vi "cm2nm_sample_organizer.vi"() -> ()   [LabVIEW 2011]
doc: "Program Purpose:\nThis program has been designed to assist with the tracking of a sample from one analytical instrument to another such as SEM, microscopes, micro x-ray diffraction and other instruments where particular positions/locations on the sample are examined, photographed, etc. The software is designed to easily enter the position of fiducials and locations of interest such that in a future session in the same of different instrument the positions of interest can be re-found through using the known location fiducials in the current and reference session to transform the point into the current sessions coordinate system. The software is dialog box driven guiding the user through the necessary data entry and program choices. Information is stored in a series of text based extensible markup language (XML) files.\n\nSome terminology used for the software:\nSample -- The item itself usually a new standard sample holder designed to have built in fiducials. \nSession -- a particular use the sample in an instrument where the sample is stationary in the instrument so the fiducials only need to be found once to associate it with reference a session. A reference session is a previous session where the fiducials and other spots of interest.\nSpots -- a location or position on the sample where data is taken as an image, spectra or other data forms applicable to analytical instruments. Note fiducials are special spots that are used as references for registering the locations from one session to another.\n\nProgram Startup:\nThe software is designed to be built into a standard windows or OS-X installer by the development platform. Once installed the program will be found under Start->Programs->cm2nm->Sample Organizer or in the OS-x Applications folder. The program will launch and show a graphical uses interface with organized into several selectable tabs. In addition there are developer information tab that will generally hidden from the users:\n• Sample Information\n• LocationDataBase\n• Current Session\n• Plots\n• Current Session Spot Text \n• Transformation Matrix [hidden from users]\nThe software is event driven and will initialize with no session loaded and the buttons to load. There are several buttons available outside the tabs that are of global use:\n• New Sample – press to start with a blank sample. Warnings should are issued about opening a new sample when an old sample may be open, giving operator an opportunity to stop and save. A dialog for entering basic sample information opens when this button is pressed.\n• Load Existing Sample – press to select an exiting sample file. A standard file system dialog box is started allowing user to select a sample file.\n• Save – ensures the current sample data base has been written to the sample file.\n• New Session with this Sample – initiates a new blank session with no spots for the current sample. The new session becomes the current session. A dialog box is started to prompt user for session information. Software will provide ample locations for user to enter notes about the session.\n• Build Date – this is a read only field to allow user to know the version of the software by build date. \n\nBasic File Structure:\n <sample>.xml [top level file that contains an array of pointers to the session data files]\n <session_n>.xml [session information with an array of spots]\n Array of spots has fields that point to files that are generated out side this program either instrument or user generated files associated with spots.\nTabs\nSample Information Tab\nThe sample information tab provides the user with an interface to get an overview of the sample including the sample name or ID and general notes on the sample. This tab has a read only field to provide the file name and path for the sample main database (XML) file. This tab also provides the ability to select a session and spot location for editing or viewing of the information about the sample. The user will use a drop down box containing the session names for the sample. When the users changes the selection on this drop down box the information displayed in the Session Information View field. Another drop down will contain the names of the spots in the selected session. When the user selects the spot the details of that spot will allows be displayed in the Information View window.\n\nLocation Data Base Tab\nThe location data base tab provides a read only overview of the session and spots associated with this sample. Session names are listed on the top row. Spot names are listed in the first column. The table shows X in the boxes at the intersection of a session and spot when a spot was recorded for that session. A C indicates that the position for that spot. The intent is an overview of the data available for the sample.\n\nCurrent Session Tab\nThe current session tab is the primary interface while a sample is in an instrument. The current session tab provides the interface to give status of the session with regards to the number of fiducials found and the current list of spots in the session. A similar view to that in the Sample Information Tab shows the general session information for the current session and the details of a spot selected with a drop down selector. A Modify button allows a user to alter the information about a selected spot through a dialog box driven process. The user is allowed to add new spots and fiducial spots at any time during the session. Another button for Find a Spot From a Previous Session becomes available only after a minimum number of three matching fiducials are first added. A Fiducial Count indicator gives feedback to the user of the number of fiducials located with the number of squares. The color of the squares indicates with yellow that not enough fiducials are been found, blue that a minimum number of fiducials have been found and green when the more than enough have been added. Each of the add spot buttons will open a dialog box to guide the user through the process of the particular type of add.\n\nPlots Tab\nThe Plots Tab will display a graphically X-Y plot of the current constellation of the spots in the current session. Only preliminary development has occurred on this user information screen to date.\n\nCurrent Session Spot Text Tab\nThe Current Session Spot Text provides a text field with a comma delimited output of the spots in the current session with the locations and names of the spots. It is intended for easy pasting into a spreadsheet.\n\nTransfomration Matrix Tab\nThe Transformation Matrix Tab is not intended for general use. It is available in the developers interface for inspection of the coordinate transformation information and a platform to generate some testing information for those."
uses:
  Sample_top_level.ctl
  Sample_Session_info.ctl
  cm2nm_sample_set.ctl
  cm2nm_coordinate_information_v2.ctl
  Instrument_type_enum_v2.ctl
  transformMatrix.ctl
  <vilib>/Analysis/Matrix/Datatypes/RealMatrix.ctl
  <vilib>/Utility/xml.llb/Read From XML File(string).vi
  <vilib>/Analysis/Matrix/NI_Matrix.lvlib
panel:
  in  "SessionIndex":i32=-1
  out "Sample Set":T1
  out "Build Date":string="July 9, 2012"
  in  "delete":bool
  out "SpotPrevSessionIndex":i32[](array[numeric])
  in  "Waiting":string
  out "SpotPrevCalcIndex":i32[](array[numeric])
  in  "Start New Session":bool
  in  "Load":bool
  in  "New Sample":bool
  in  "Save Sample Information":bool
  out "subarray":string[](array[string])
  out "Label.Text":string="CollectionOfPoints"
  in  "Tab Control":T4(tab)
  in  "Sessions For This Sample.":u16(ring) items=["FEI_initial", "jill_redo", "fixing_jill_fid5", "try_fix_5again"]
  out "Sample Information":T5={"Sample Name/ID"="", "Notes on Sample"="", "Session_list"=[{"Instrument"=2, "Session_data_base"=path "/INL Macintosh/Users/timothymcjunkin/Desktop/Diffusion couple/JEOL 7000F SEM 9-3-10/Jeol_9-3-10.xml", "Session Name/ID"="Initial Joel location"}, {"Instrument"=3, "Session_data_base"=path "/INL Macintosh/Users/timothymcjunkin/Desktop/Diffusion couple/MXRD 9-13-10/xrd_session.xlm", "Session Name/ID"="xrd_test"}, {"Instrument"=2, "Session_data_base"=path "/INL Macintosh/Users/timothymcjunkin/Desktop/Diffusion couple/JEOL 7000F SEM 9-3-10/Corrected_9-3-10.xlm", "Session Name/ID"="Correct_Abs_position"}]} {"Session_list"."Instrument" items=["Unknown", "Phillips SEM IRC", "JEOL 7000F EML_MFC", "MXRD MFC", "JEOL_EPMA"]}
  out "Sample_data_base":path
  out "Session Information View":T1={"CollectionOfPoints"=[{"MetaDataFile"=path "", "X"=0.0, "Y"=0.0, "Z"=0.0, "Group"=0, "Rotation"=0.0, "Fiducial"=FALSE, "Magnification"=0.0, "Working_Distance"=0.0, "Notes"="", "Location Name/ID"="", "OtherRelatedDataFiles"=[], "Available"=FALSE}, {"MetaDataFile"=path "", "X"=0.0, "Y"=0.0, "Z"=0.0, "Group"=0, "Rotation"=0.0, "Fiducial"=FALSE, "Magnification"=0.0, "Working_Distance"=0.0, "Notes"="", "Location Name/ID"="", "OtherRelatedDataFiles"=[], "Available"=FALSE}, {"MetaDataFile"=path "", "X"=0.0, "Y"=0.0, "Z"=0.0, "Group"=0, "Rotation"=0.0, "Fiducial"=FALSE, "Magnification"=0.0, "Working_Distance"=0.0, "Notes"="", "Location Name/ID"="", "OtherRelatedDataFiles"=[], "Available"=FALSE}, {"MetaDataFile"=path "", "X"=0.0, "Y"=0.0, "Z"=0.0, "Group"=0, "Rotation"=0.0, "Fiducial"=FALSE, "Magnification"=0.0, "Working_Distance"=0.0, "Notes"="", "Location Name/ID"="", "OtherRelatedDataFiles"=[], "Available"=FALSE}, {"MetaDataFile"=path "", "X"=0.0, "Y"=0.0, "Z"=0.0, "Group"=0, "Rotation"=0.0, "Fiducial"=FALSE, "Magnification"=0.0, "Working_Distance"=0.0, "Notes"="", "Location Name/ID"="", "OtherRelatedDataFiles"=[], "Available"=FALSE}, {"MetaDataFile"=path "", "X"=0.0, "Y"=0.0, "Z"=0.0, "Group"=0, "Rotation"=0.0, "Fiducial"=FALSE, "Magnification"=0.0, "Working_Distance"=0.0, "Notes"="", "Location Name/ID"="", "OtherRelatedDataFiles"=[], "Available"=FALSE}], "Instrument"=enum."JEOL 7000F EML_MFC", "CollectionFile"=path "/INL Macintosh/Users/timothymcjunkin/Desktop/Diffusion couple/JEOL 7000F SEM 9-3-10/Corrected_9-3-10.xlm", "Session Name/ID"="Correct_Abs_position", "SessionNotes"="EMSA images were taken off center so I May need to add the two together"}
  in  "Spots For Selected Session":u16(ring) items=["Fid1", "Fid2", "Fid3", "Fid4", "Fid5", "point1", "Interface_to_fosil", "on_fosil_1", "Fid4-as_calculated", "Fid2-alt-as-calculated", "point1-alt-ascalculated"]
  in  "Edit Spot":bool
  out "Cluster":T2
  in  "Sample locations of Interest":string[][](table)
  in  "modify":bool
  in  "Add Fiducial":bool
  in  "Add_spots":bool
  in  "Batch Add MetaDataFiles":bool
  in  "Spots Current Session":u16(ring) items=["Fid1", "Fid3", "Fid5", "Fid2", "Fid4", "point1", "zalt_calc_Fid2-alt", "zalt_calc_Fid4-alt", "zalt_ascalc_point1-alt"]
  out "Fiducial Count":u32[](array[colorbox])=[3071, 3071, 3071]
  out "Current Session View":T1={"CollectionOfPoints"=[{"MetaDataFile"=path "", "X"=0.0, "Y"=0.0, "Z"=0.0, "Group"=0, "Rotation"=0.0, "Fiducial"=FALSE, "Magnification"=0.0, "Working_Distance"=0.0, "Notes"="", "Location Name/ID"="", "OtherRelatedDataFiles"=[], "Available"=FALSE}, {"MetaDataFile"=path "", "X"=0.0, "Y"=0.0, "Z"=0.0, "Group"=0, "Rotation"=0.0, "Fiducial"=FALSE, "Magnification"=0.0, "Working_Distance"=0.0, "Notes"="", "Location Name/ID"="", "OtherRelatedDataFiles"=[], "Available"=FALSE}, {"MetaDataFile"=path "", "X"=0.0, "Y"=0.0, "Z"=0.0, "Group"=0, "Rotation"=0.0, "Fiducial"=FALSE, "Magnification"=0.0, "Working_Distance"=0.0, "Notes"="", "Location Name/ID"="", "OtherRelatedDataFiles"=[], "Available"=FALSE}, {"MetaDataFile"=path "", "X"=0.0, "Y"=0.0, "Z"=0.0, "Group"=0, "Rotation"=0.0, "Fiducial"=FALSE, "Magnification"=0.0, "Working_Distance"=0.0, "Notes"="", "Location Name/ID"="", "OtherRelatedDataFiles"=[], "Available"=FALSE}, {"MetaDataFile"=path "", "X"=0.0, "Y"=0.0, "Z"=0.0, "Group"=0, "Rotation"=0.0, "Fiducial"=FALSE, "Magnification"=0.0, "Working_Distance"=0.0, "Notes"="", "Location Name/ID"="", "OtherRelatedDataFiles"=[], "Available"=FALSE}, {"MetaDataFile"=path "", "X"=0.0, "Y"=0.0, "Z"=0.0, "Group"=0, "Rotation"=0.0, "Fiducial"=FALSE, "Magnification"=0.0, "Working_Distance"=0.0, "Notes"="", "Location Name/ID"="", "OtherRelatedDataFiles"=[], "Available"=FALSE}, {"MetaDataFile"=path "", "X"=0.0, "Y"=0.0, "Z"=0.0, "Group"=0, "Rotation"=0.0, "Fiducial"=FALSE, "Magnification"=0.0, "Working_Distance"=0.0, "Notes"="", "Location Name/ID"="", "OtherRelatedDataFiles"=[], "Available"=FALSE}], "Instrument"=enum."MXRD MFC", "CollectionFile"=path "/INL Macintosh/Users/timothymcjunkin/Desktop/Diffusion couple/MXRD 9-13-10/xrd_session_for_corrected.xml", "Session Name/ID"="xrd_test", "SessionNotes"="Sample moved to XRD"}
  in  "Add New Spot To Session":bool
  in  "Calc Trans":bool
  out "current selection group":i32
  out "CurrentRefSessionIdx":i32
  out "FidcucialMetrics":cluster{"M1":dbl, "M2":dbl, "S1":dbl, "S2":dbl}
  in  "Plot":bool
  out "Spots in Current Session":cluster{dbl[], dbl[]}[](graph)
  out "current_transformation_matrices":T7
  in  "Sessions Spot Transform":u16(ring) items=["FEI_initial", "jill_redo", "fixing_jill_fid5", "try_fix_5again"]
  in  "NewSession_from_previous":bool
  out "ReferenceSession":T1={"CollectionOfPoints"=[{"MetaDataFile"=path "", "X"=0.0, "Y"=0.0, "Z"=0.0, "Group"=0, "Rotation"=0.0, "Fiducial"=FALSE, "Magnification"=0.0, "Working_Distance"=0.0, "Notes"="", "Location Name/ID"="", "OtherRelatedDataFiles"=[], "Available"=FALSE}, {"MetaDataFile"=path "", "X"=0.0, "Y"=0.0, "Z"=0.0, "Group"=0, "Rotation"=0.0, "Fiducial"=FALSE, "Magnification"=0.0, "Working_Distance"=0.0, "Notes"="", "Location Name/ID"="", "OtherRelatedDataFiles"=[], "Available"=FALSE}, {"MetaDataFile"=path "", "X"=0.0, "Y"=0.0, "Z"=0.0, "Group"=0, "Rotation"=0.0, "Fiducial"=FALSE, "Magnification"=0.0, "Working_Distance"=0.0, "Notes"="", "Location Name/ID"="", "OtherRelatedDataFiles"=[], "Available"=FALSE}, {"MetaDataFile"=path "", "X"=0.0, "Y"=0.0, "Z"=0.0, "Group"=0, "Rotation"=0.0, "Fiducial"=FALSE, "Magnification"=0.0, "Working_Distance"=0.0, "Notes"="", "Location Name/ID"="", "OtherRelatedDataFiles"=[], "Available"=FALSE}, {"MetaDataFile"=path "", "X"=0.0, "Y"=0.0, "Z"=0.0, "Group"=0, "Rotation"=0.0, "Fiducial"=FALSE, "Magnification"=0.0, "Working_Distance"=0.0, "Notes"="", "Location Name/ID"="", "OtherRelatedDataFiles"=[], "Available"=FALSE}, {"MetaDataFile"=path "", "X"=0.0, "Y"=0.0, "Z"=0.0, "Group"=0, "Rotation"=0.0, "Fiducial"=FALSE, "Magnification"=0.0, "Working_Distance"=0.0, "Notes"="", "Location Name/ID"="", "OtherRelatedDataFiles"=[], "Available"=FALSE}], "Instrument"=enum."JEOL 7000F EML_MFC", "CollectionFile"=path "/INL Macintosh/Users/timothymcjunkin/Desktop/Diffusion couple/JEOL 7000F SEM 9-3-10/Corrected_9-3-10.xlm", "Session Name/ID"="Correct_Abs_position", "SessionNotes"="EMSA images were taken off center so I May need to add the two together"}
  out "TransformSession Name/ID":string="Correct_Abs_position"
  out "PairedFiducialNames":T9(array[cluster])=[{"Location Name/ID"="F1", "Location Name/ID"="F1"}, {"Location Name/ID"="F3B", "Location Name/ID"="F3B"}, {"Location Name/ID"="F5C", "Location Name/ID"="F5C"}]
  out "error out 3":errorcluster
  out "error out 4":errorcluster
  in  "Sessions Spot calc From":u16(ring) items=["FEI_initial", "jill_redo", "fixing_jill_fid5", "try_fix_5again"]
  in  "Create a Report":bool
  out "Selected_Session_spots":string
  out "Current_Session_points":string
  out "concatenated string":string
  in  "FindAllSpotsFromPrevSession":bool
  in  "Data Base Directory":path=path "/INL Macintosh/Users/timothymcjunkin/Desktop/diff_couple"
  in  "Enter New Location/Position":T2
  in  "Transform a Pnt.":bool
  in  "Get Coords":bool
  in  "LoadSessionIntoCurrent":bool
  out "error out 2":errorcluster caption="error out"
  out "CurrentSessionOut":T2[](array[typedef])
  out "Array":bool[](array[boolean])
  out "Index Values":u32[](array[numeric])=[2]
  in  "stop":bool
  # "Sessions"
  # "Sample Spots"
  # "X indicates an entered (presumably confirmed point)\nc indicates a calculated position."
  # "Selected spot can be  viewed  or modified \nin the information on the right"
  # "This now contains spots found in this session.\nSpots with only pre-calculated positions are\naccessed with \"Find A Spot From A Previous\nSession\" Button."
  # "for debug only"
  # "NF = not fiducial"
  # "Calcualted means\ntransformed from\nprevious session\nConfirmed has\nbeen found during\ncurrent session."
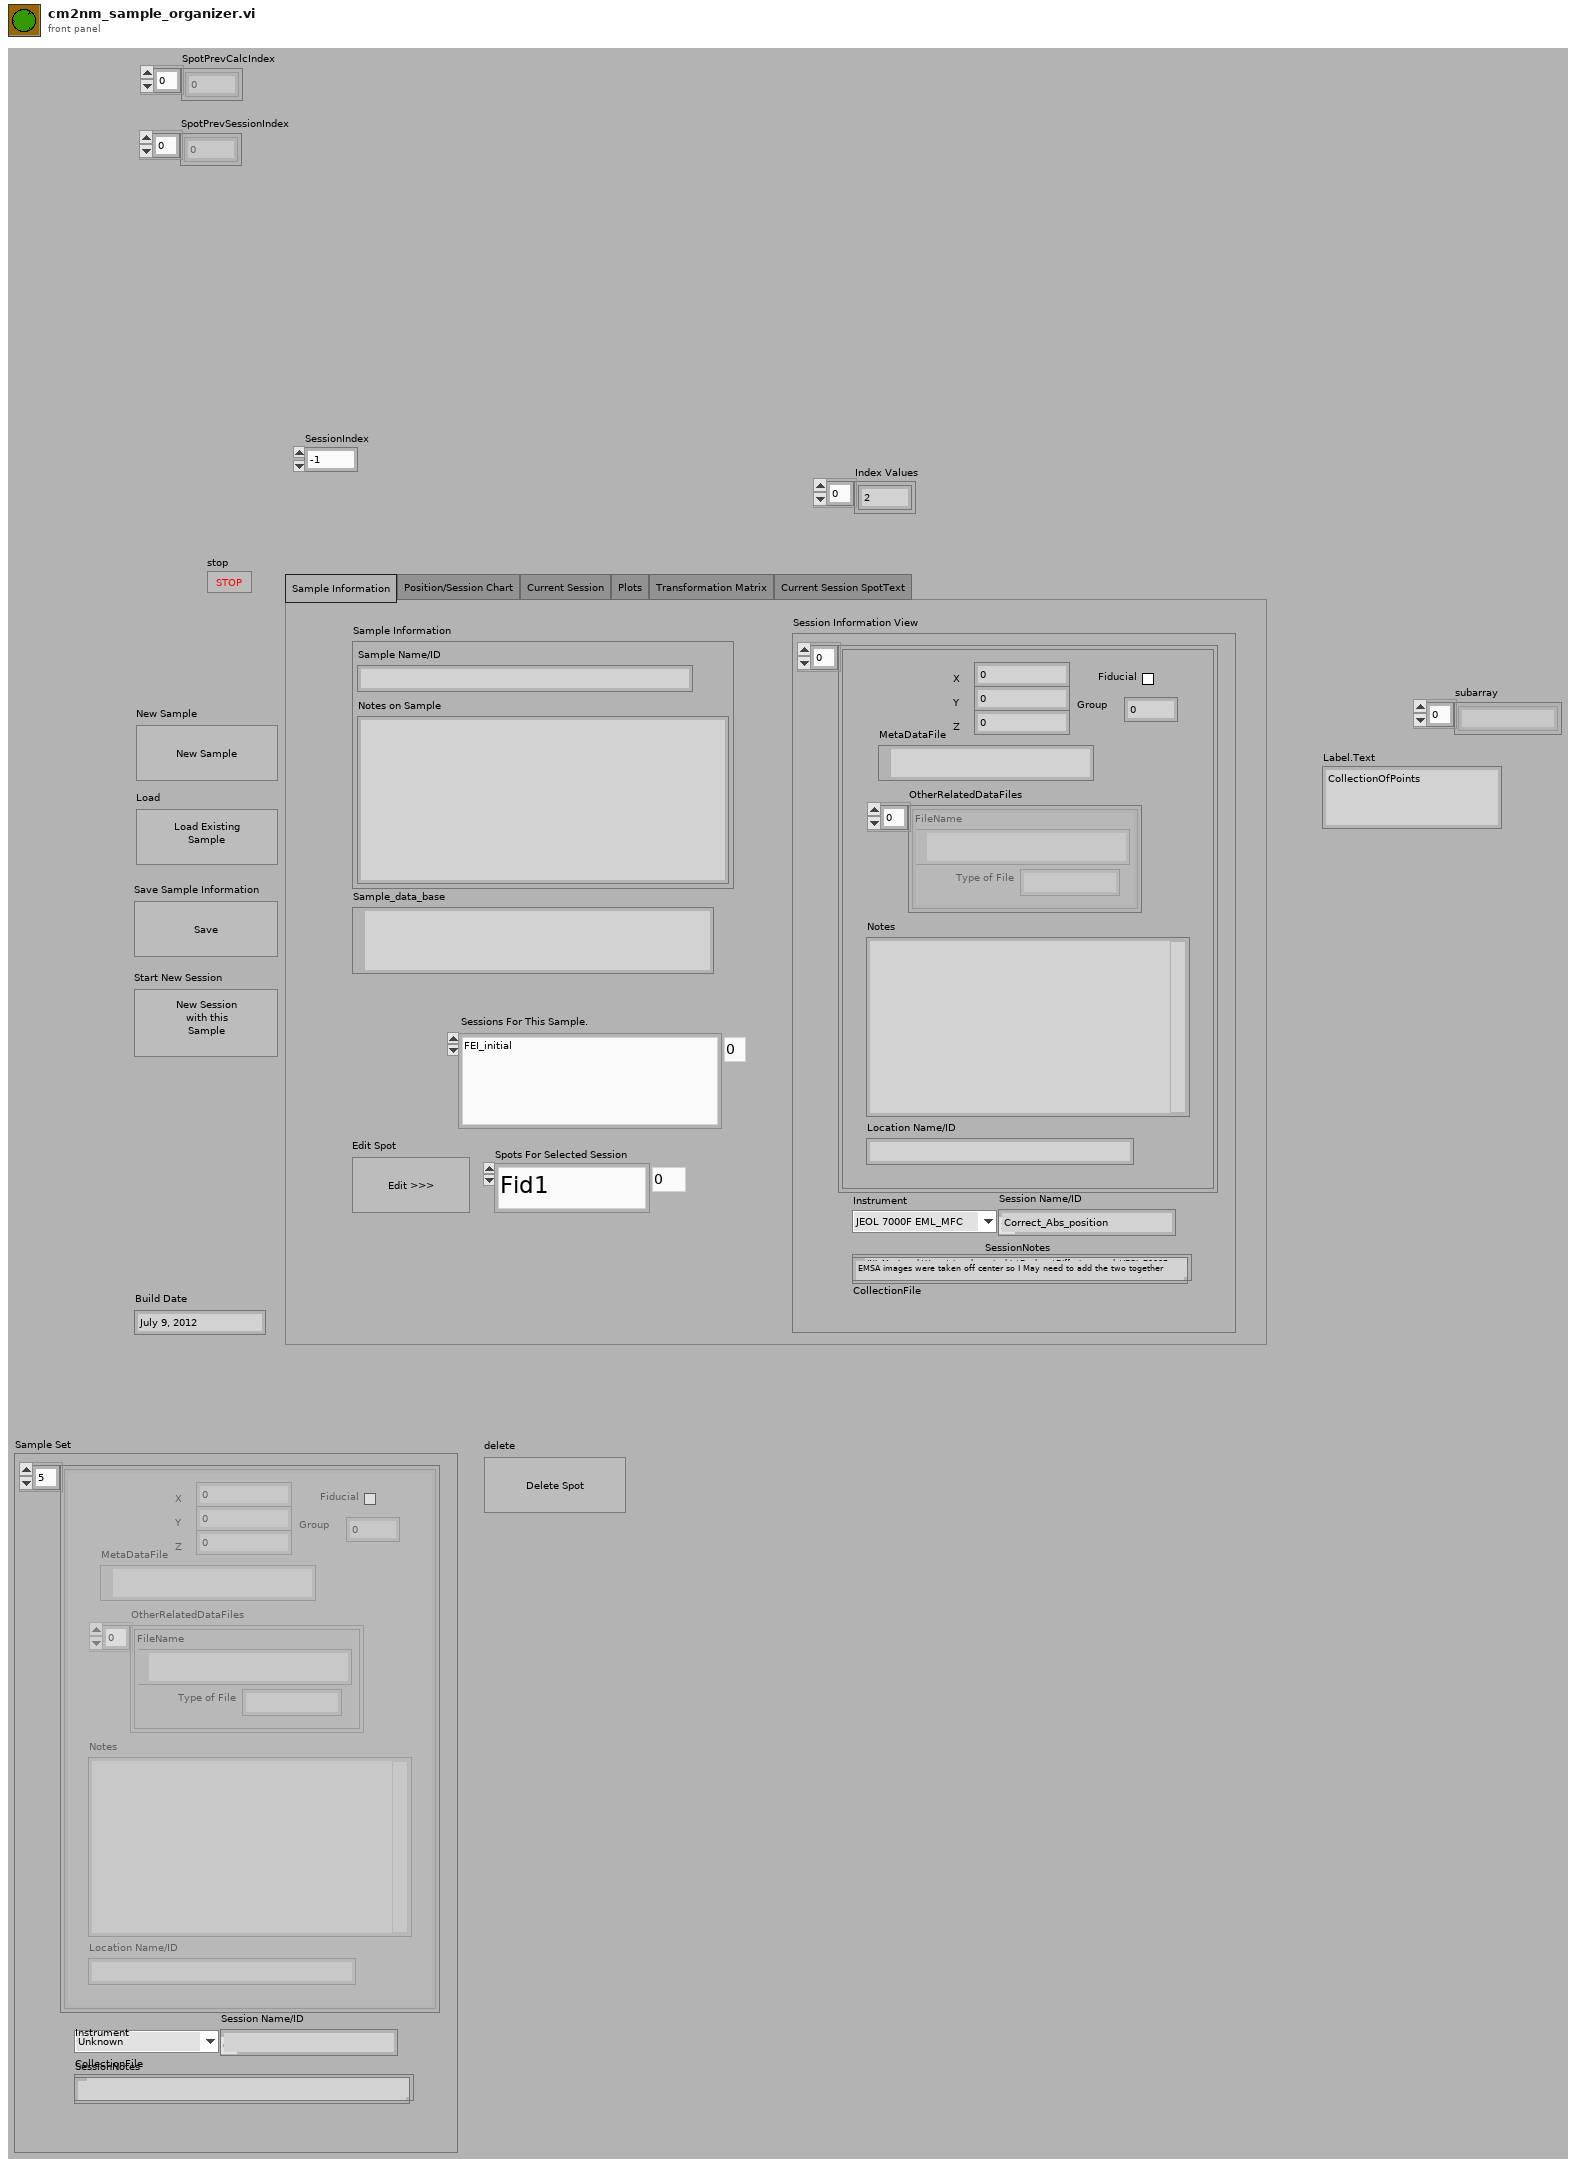
[diagram p1: front panel]
types:
  T1 = typedef "cm2nm_sample_set.ctl" = cluster{"CollectionOfPoints":T2[], "Instrument":T3, "CollectionFile":path, "Session Name/ID":string, "SessionNotes":string}
  T2 = typedef "cm2nm_coordinate_information_v2.ctl" = cluster{"MetaDataFile":path, "X":dbl, "Y":dbl, "Z":dbl, "Group":i32, "Rotation":dbl[unit], "Fiducial":bool, "Magnification":dbl, "Working_Distance":dbl, "Notes":string, "Location Name/ID":string, "OtherRelatedDataFiles":cluster{"Type of File":string, "FileName":path}[], "Available":bool}
  T3 = typedef "Instrument_type_enum_v2.ctl" = enum16{"Unknown", "Philips FEI SEM IRC", "JEOL 7000F EML_MFC", "MXRD MFC", "JEOL_EPMA"}
  T4 = enum32{"Sample Information", "Position/Session Chart", "Current Session", "Plots", "Transformation Matrix", "Current Session SpotText", "Extras"}
  T5 = typedef "Sample_top_level.ctl" = cluster{"Sample Name/ID":string, "Notes on Sample":string, "Session_list":T6[]}
  T6 = typedef "Sample_Session_info.ctl" = cluster{"Instrument":u16, "Session_data_base":path, "Session Name/ID":string}
  T7 = typedef "transformMatrix.ctl" = cluster{"A":T8, "B":T8, "C":T8}
  T8 = typedef "NI_Matrix.lvlib/RealMatrix.ctl" = dbl[][]
  T9 = cluster{"Location Name/ID":string, "Location Name/ID":string}[]
  T10 = enum8{"Enabled", "Disabled", "Disabled and Grayed Out"}
  T11 = cluster{"CollectionOfPoints":T2[], "Instrument":u16, "CollectionFile":path, "Session Name/ID":string, "SessionNotes":string}
  T12 = cluster{"Sample Name/ID":string, "Notes on Sample":string, "Session_list":cluster{"Instrument":u16, "Session_data_base":path, "Session Name/ID":string}[]}
  T13 = cluster{"Instrument":u16, "Session_data_base":path, "Session Name/ID":string}
  T14 = cluster{"Instrument":u16, "Session_data_base":path, "Session Name/ID":string}[]
  T15 = typedef "cm2nm_sample_set.ctl" = cluster{"CollectionOfPoints":T16[], "Instrument":u16, "CollectionFile":path, "Session Name/ID":string, "SessionNotes":string}
  T16 = typedef "cm2nm_coordinate_information_v2.ctl" = cluster{"MetaDataFile":path, "X":dbl, "Y":dbl, "Group":i32, "Z":dbl, "Rotation":dbl[unit], "Fiducial":bool, "Magnification":dbl, "Working_Distance":dbl, "Notes":string, "Location Name/ID":string, "OtherRelatedDataFiles":cluster{"Type of File":string, "FileName":path}[], "Available":bool}
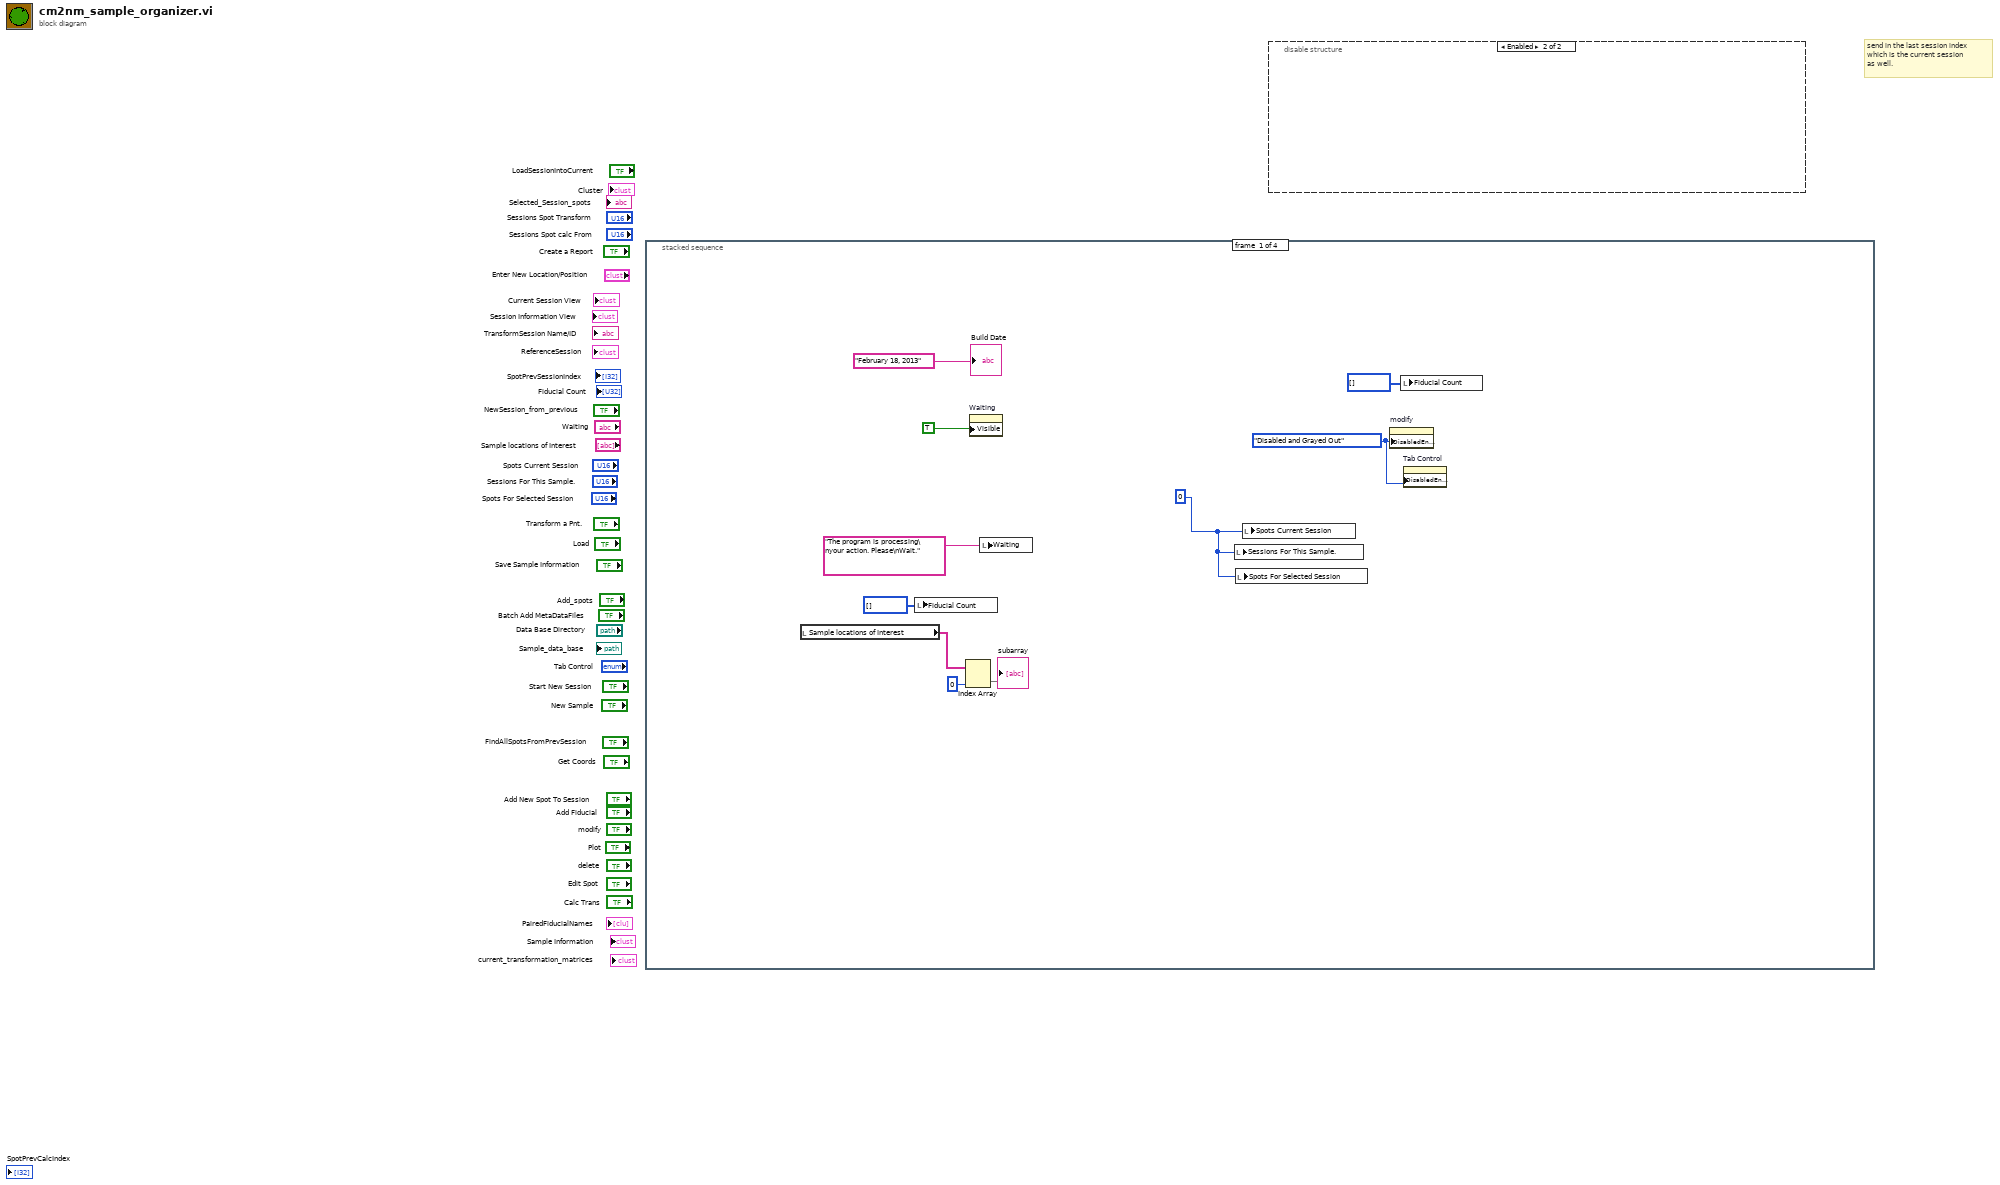
[diagram p0: block diagram]
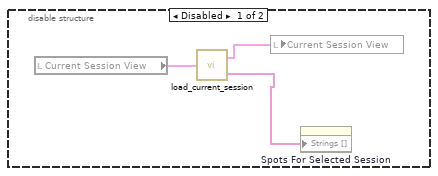
[diagram p2: hidden frame]
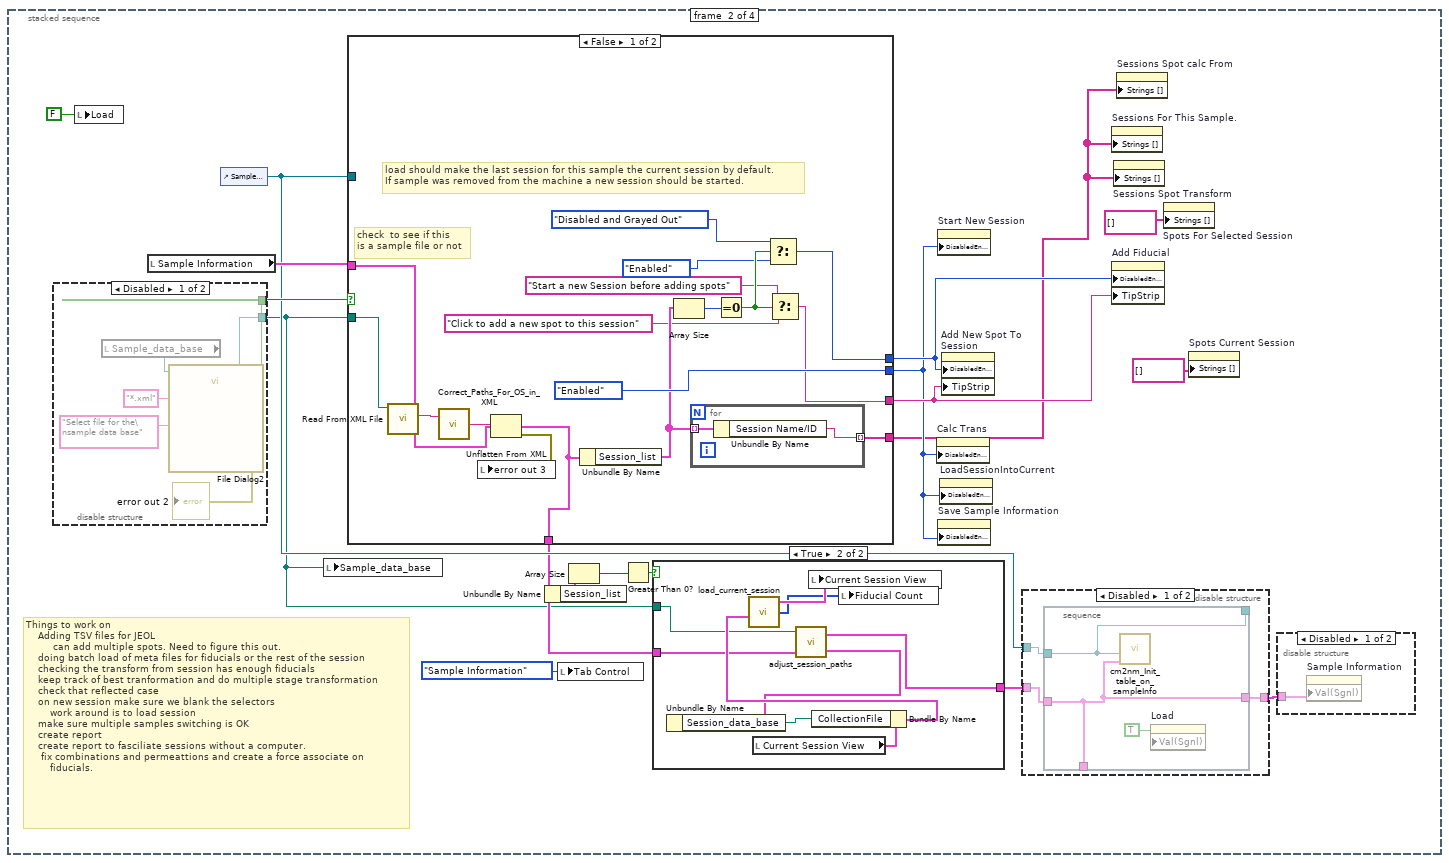
[diagram p3: hidden frame]
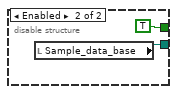
[diagram p6: hidden frame]
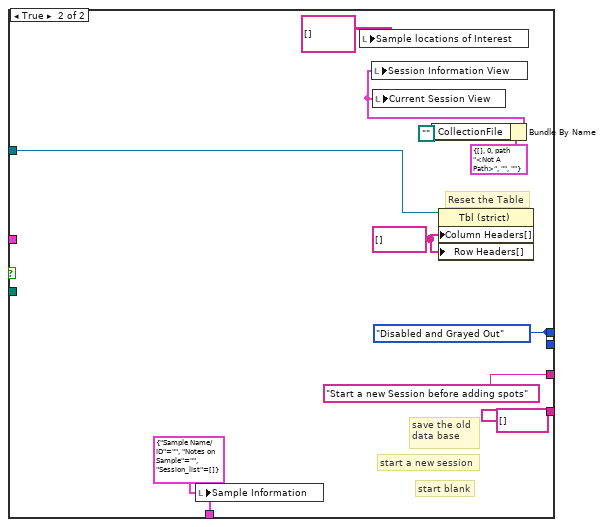
[diagram p8: hidden frame]
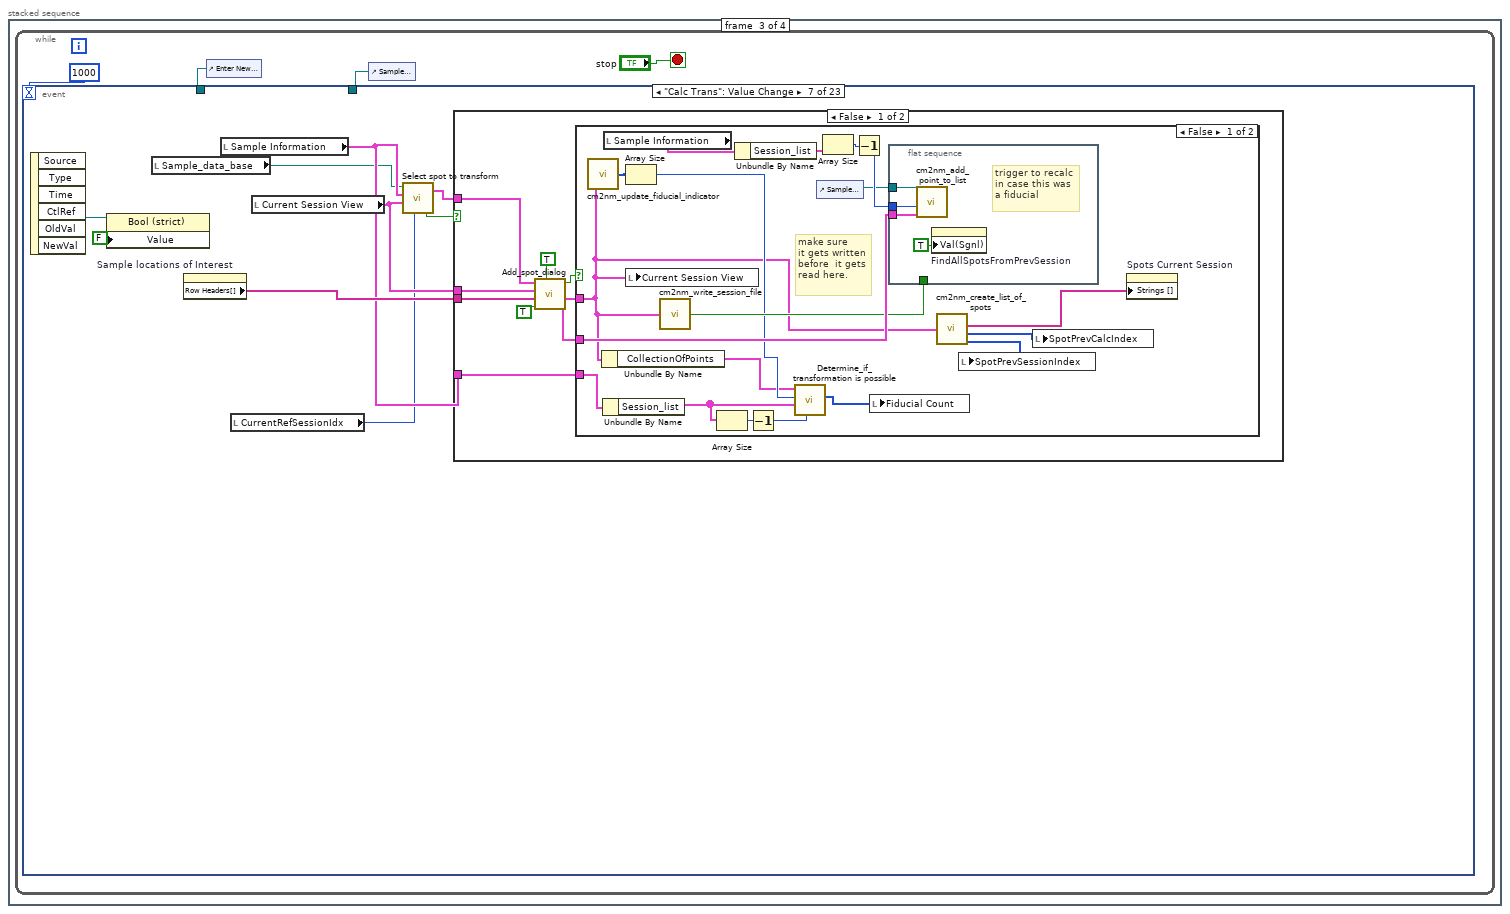
[diagram p9: hidden frame]
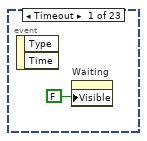
[diagram p10: hidden frame]
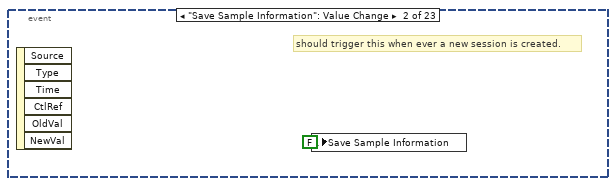
[diagram p11: hidden frame]
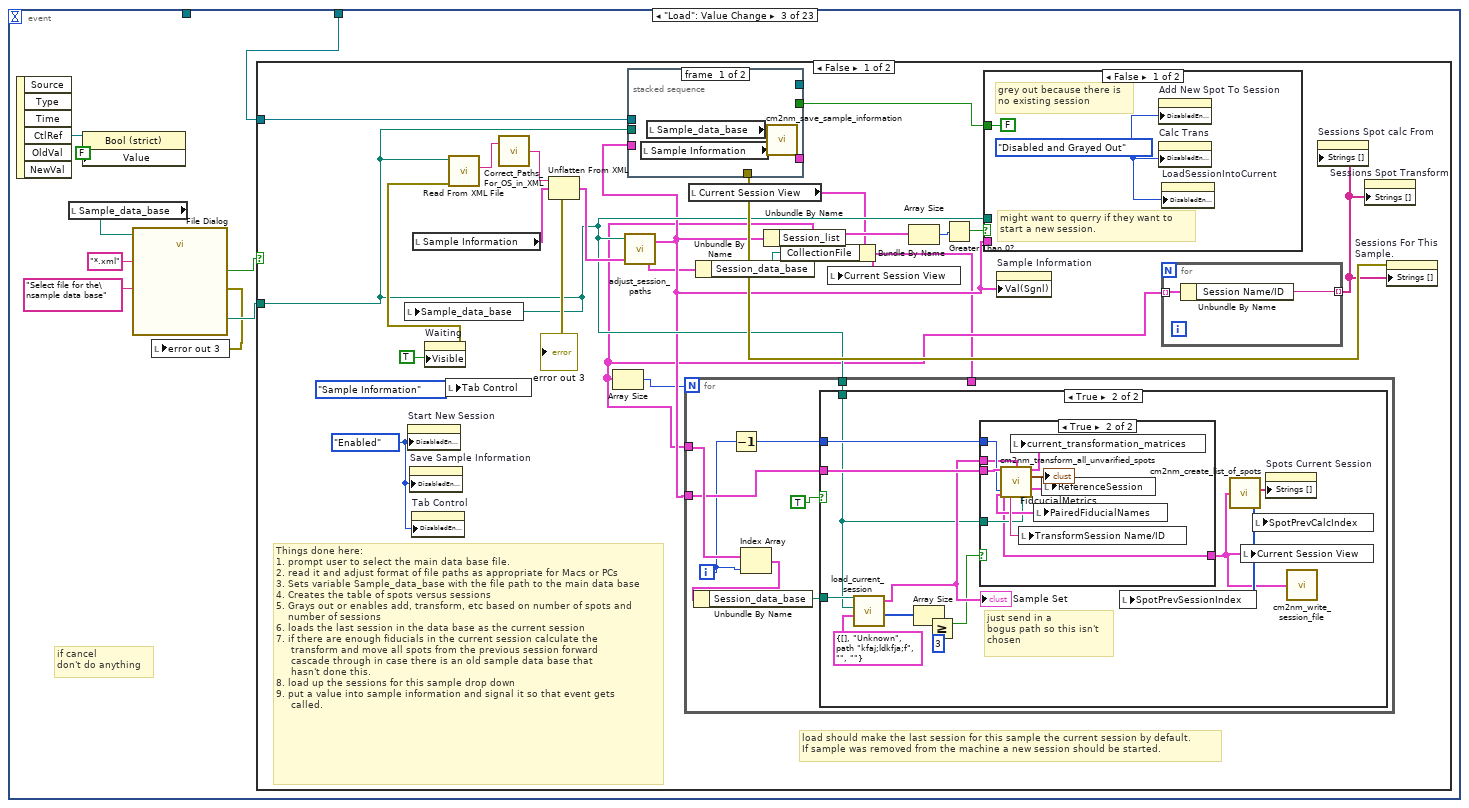
[diagram p12: hidden frame]
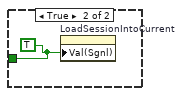
[diagram p15: hidden frame]
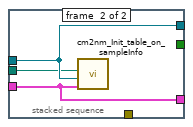
[diagram p16: hidden frame]
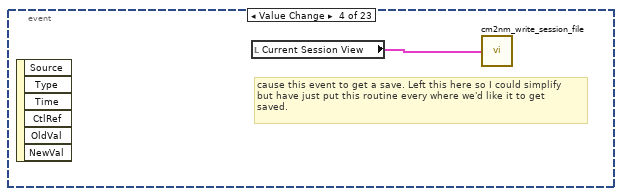
[diagram p18: hidden frame]
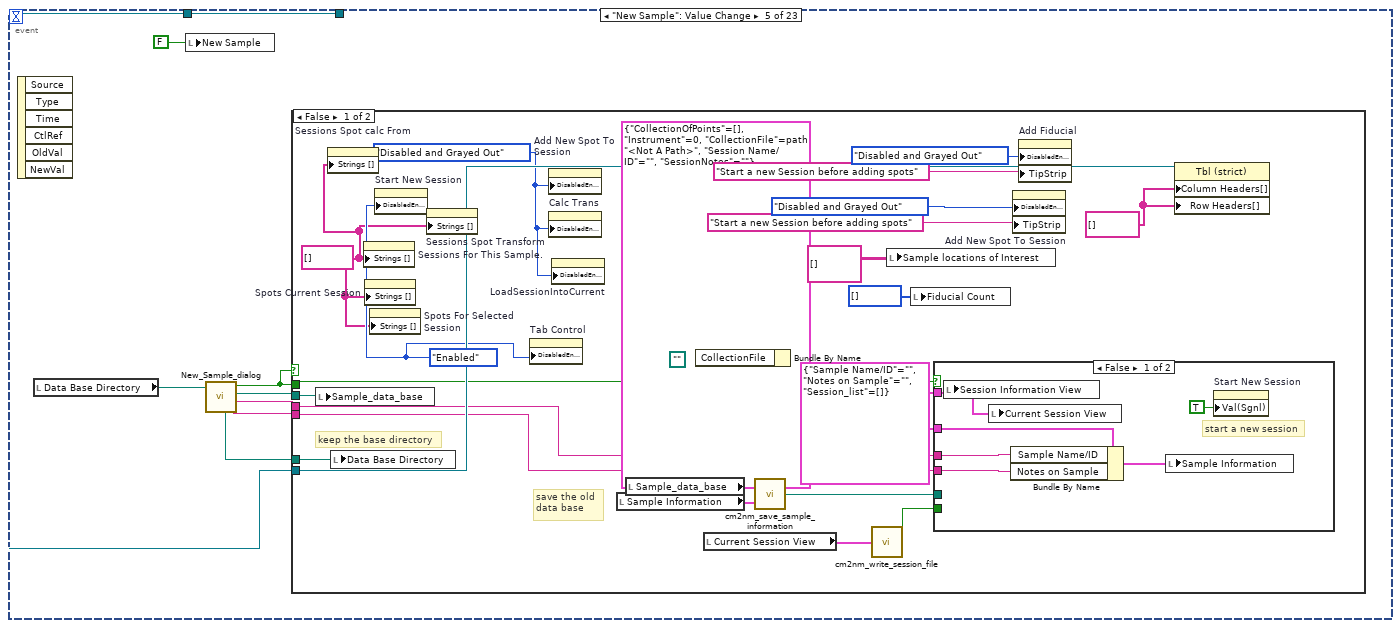
[diagram p19: hidden frame]
diagram:
  # "send in the last session index\nwhich is the current session\nas well."
  n1 = stacked-sequence {
    frame #0 {
      w7 = 0
      w5 = T10."Disabled and Grayed Out" ("Disabled")
      n2 = local read "Sample locations of Interest"() -> (w2:string[][])
      n3 = local write "Fiducial Count"(u32[] [] ("Fiducial Count")) -> ()
      n4 = Index Array(array=w2, index (col)=0 ("disabled index (col)")) -> (element=→"subarray":string[])  [unwired: 1 in]
      n5 = property on="Waiting" class="Str"("Visible"=TRUE) -> ()  [unwired: 2 in, 2 out]
      n6 = local write "Waiting"("The program is processing\nyour action. Please\nWait." ("Waiting")) -> ()
      n7 = local write "Sessions For This Sample."(w7) -> ()
      n8 = local write "Spots For Selected Session"(w7) -> ()
      n9 = local write "Spots Current Session"(w7) -> ()
      n10 = property on="modify" class="Bool (strict)"("DisabledEnum"=w5) -> ()  [unwired: 2 in, 2 out]
      n11 = local write "Fiducial Count"(u32[] [] ("Fiducial Count")) -> ()
      n12 = property on="Tab Control" class="TabCtl (strict)"("DisabledEnum"=w5) -> ()  [unwired: 2 in, 2 out]
      "Build Date" <- "February 18, 2013" ("Build Date")
    }
    frame #1 {
      # "Things to work on\n    Adding TSV files for JEOL\n         can add multiple spots. Need to figure this out.\n    doing batch load of meta files for fiducials or the rest of the session\n    checking the transform from session has enough fiducials\n    keep track of best tranformation and do multiple stage transformation\n    check that reflected case\n    on new session make sure we blank the selectors\n        work around is to load session\n    make sure multiple samples switching is OK\n    create report\n    create report to fasciliate sessions without a computer. \n     fix combinations and permeattions and create a force associate on\n        fiducials."
      n13 = disable-structure shown="Disabled" {
        disable-tunnel: [w41 TRUE ("cancelled")] -> w27
        disable-tunnel: [w37 w42] -> w11
        frame Disabled {
          n14 = local read "Sample_data_base"() -> (w40:path)
          n15 = call "File Dialog2"("start path"=w40, "prompt"="Select file for the\nsample data base", "pattern (all files)"="*.xml") -> ("selected path"=w37:path, "cancelled"=w41:bool, "error out"=→"error out 2":errorcluster)  [unwired: 9 in, 1 out]
        }
        frame Enabled {
          n16 = local read "Sample_data_base"() -> (w42:path)
        }
      }
      n17 = local write "Load"(FALSE ("Load")) -> ()
      n18 = local read "Sample Information"() -> (w24:T5)
      n19 = control-ref of="Sample locations of Interest"() -> (w22:refnum<vi>)
      n20 = local write "Sample_data_base"(w11) -> ()
      n21 = case shown="False" w27 {
        tunnel: w22 -> [_ w76]
        tunnel: w11 -> [w70 _]
        tunnel: w24 -> [w69 _]
        tunnel: [w54 w75] -> w20
        tunnel: [T10."Enabled" ("Disabled") w74] -> w16
        tunnel: [w66 string[] [] ("Strings []")] -> w12
        tunnel: [w59 w74] -> w18
        tunnel: [w58 "Start a new Session before adding spots" ("Tip Strip")] -> w17
        frame False {
          # "check  to see if this\nis a sample file or not"
          # "load should make the last session for this sample the current session by default.\nIf sample was removed from the machine a new session should be started."
          n22 = call-poly <vilib>:"Read From XML File.vi"("XML File Path"=w70) -> ("XML Elements"=w68:string)  [unwired: 1 in, 9 out]
          n23 = call "Correct_Paths_For_OS_in_XML.vi"("XML Elements"=w68) -> ("String"=w67:string)  [unwired: 1 in]
          n24 = Unflatten From XML(xml string=w67, type=w69) -> (value=w54:T5, error out=w55:errorcluster)  [unwired: 1 in]
          n25 = local write "error out 3"(w55) -> ()
          n26 = Unbundle By Name(w54) -> ("Session_list"=w64:T6[])
          n27 = Array Size(array=w64) -> (size(s)=w63:i32)
          n28 = for {
            tunnel: w64 -> [w72] mode=indexing
            tunnel: [w71] -> w66 mode=indexing
            n29 = Unbundle By Name(w72) -> ("Session Name/ID"=w71:string)
          }
          n30 = Equal To 0?(x=w63) -> (x = 0?=w62:bool)
          n31 = Select(t=T10."Disabled and Grayed Out" ("Disabled"), s=w62, f=T10."Enabled" ("Disabled")) -> (s? t:f=w59:T10)
          n32 = Select(t="Start a new Session before adding spots" ("Tip Strip"), s=w62, f="Click to add a new spot to this session" ("Tip Strip")) -> (s? t:f=w58:string)
        }
        frame True {
          w74 = T10."Disabled and Grayed Out" ("Disabled")
          w82 = string[] [] ("Column Header Strings[]")
          w75 = T12 {"Sample Name/ID"="", "Notes on Sample"="", "Session_list"=[]} ("Sample_Information")
          # "start blank"
          # "start a new session"
          # "save the old \ndata base"
          # "Reset the Table"
          n33 = local write "Sample Information"(w75) -> ()
          n34 = local write "Sample locations of Interest"(string[][] [] ("Sample locations of Interest")) -> ()
          n35 = Bundle By Name(cluster=T11 {"CollectionOfPoints"=[], "Instrument"=0, "CollectionFile"=path "<Not A Path>", "Session Name/ID"="", "SessionNotes"=""} ("Sample Set"), "CollectionFile"=path "") -> (w78:T11)
          n36 = local write "Session Information View"(w78) -> ()
          n37 = local write "Current Session View"(w78) -> ()
          n38 = property on="Property Node" class="Tbl (strict)"(reference=w76, "Column Headers[]"=w82, "Row Headers[]"=w82) -> ()  [unwired: 1 in, 2 out]
        }
      }
      n39 = Unbundle By Name(w20) -> ("Session_list"=w21:T6[])
      n40 = local write "Tab Control"(T4."Sample Information" ("Tab Control")) -> ()
      n41 = Array Size(array=w21) -> (size(s)=w26:i32)
      n42 = Greater Than 0?(x=w26) -> (x > 0?=w25:bool)
      n43 = case shown="True" w25 {
        tunnel: w11 -> [_ w48]
        tunnel: w20 -> [w44 w47]
        tunnel: [w44 w46] -> w23
        frame False {
        }
        frame True {
          n44 = local read "Current Session View"() -> (w53:T1)
          n45 = call "adjust_session_paths.vi"("Sample_Information In"=w47, "top_level"=w48) -> ("MostRecentSessionOut"=w49:T13, "Sample_Information_out"=w46:T12)  [unwired: 1 in]
          n46 = Unbundle By Name(w49) -> ("Session_data_base"=w52:path)
          n47 = Bundle By Name(cluster=w53, "CollectionFile"=w52) -> (w50:T1)
          n48 = call "load_current_session.vi"("Current Session Information"=w50) -> ("Fiducial Count"=w45:u32[], "Sample Set"=w51:T1)  [unwired: 3 in, 1 out]
          n49 = local write "Current Session View"(w51) -> ()
          n50 = local write "Fiducial Count"(w45) -> ()
        }
      }
      n51 = property on="Calc Trans" class="Bool (strict)"("DisabledEnum"=w16) -> ()  [unwired: 2 in, 2 out]
      n52 = property on="Start New Session" class="Bool (strict)"("DisabledEnum"=w16) -> ()  [unwired: 2 in, 2 out]
      n53 = property on="Save Sample Information" class="Bool (strict)"("DisabledEnum"=w16) -> ()  [unwired: 2 in, 2 out]
      n54 = property on="LoadSessionIntoCurrent" class="Bool (strict)"("DisabledEnum"=w16) -> ()  [unwired: 2 in, 2 out]
      n55 = property on="Add New Spot To Session" class="Bool (strict)"("DisabledEnum"=w18, "TipStrip"=w17) -> ()  [unwired: 2 in, 2 out]
      n56 = disable-structure shown="Disabled" {
        disable-tunnel: w23 -> [w31 _]
        disable-tunnel: w22 -> [w30 _]
        disable-tunnel: [w29 _] -> w19
        frame Disabled {
          n57 = stacked-sequence {
            tunnel: w31 -> [w33]
            tunnel: w30 -> [w34]
            tunnel: [w34] -> _
            tunnel: [w33] -> _
            tunnel: [w33] -> w29
            frame #0 {
              n58 = call "cm2nm_Init_table_on_sampleInfo.vi"("Sample_Information"=w33, "Sample locations of Interest"=w34) -> ()  [unwired: 1 in, 3 out]
              n59 = property on="Load" class="Bool (strict)"("Val(Sgnl)"=TRUE ("Value (Signaling)")) -> ()  [unwired: 2 in, 2 out]
            }
          }
        }
        frame Enabled {
        }
      }
      n60 = property on="Sessions For This Sample." class="Ring (strict)"("Strings []"=w12) -> ()  [unwired: 2 in, 2 out]
      n61 = property on="Add Fiducial" class="Bool (strict)"("DisabledEnum"=w18, "TipStrip"=w17) -> ()  [unwired: 2 in, 2 out]
      n62 = property on="Sessions Spot Transform" class="Ring (strict)"("Strings []"=w12) -> ()  [unwired: 2 in, 2 out]
      n63 = property on="Sessions Spot calc From" class="Ring (strict)"("Strings []"=w12) -> ()  [unwired: 2 in, 2 out]
      n64 = property on="Spots For Selected Session" class="Ring (strict)"("Strings []"=string[] []) -> ()  [unwired: 2 in, 2 out]
      n65 = property on="Spots Current Session" class="Ring (strict)"("Strings []"=string[] [] ("Array")) -> ()  [unwired: 2 in, 2 out]
      n66 = disable-structure shown="Disabled" {
        disable-tunnel: w19 -> [w35 _]
        frame Disabled {
          n67 = property on="Sample Information" class="Clust (strict)"("Val(Sgnl)"=w35) -> ()  [unwired: 2 in, 2 out]
        }
        frame Enabled {
        }
      }
    }
    frame #2 {
      n68 = while {
        stop <- "stop" stop-if-true
        n69 = control-ref of="Enter New Location/Position"() -> (w83:refnum<vi>)
        n70 = control-ref of="Sample locations of Interest"() -> (w85:refnum<vi>)
        n71 = event shown="[6] \"Calc Trans\": Value Change" {
          selector: _ -> [_ _ _ _ _ _ _ _ _ _ _ _ _ _ _ _ _ _ _ _ _ _ _]
          dyn-events: _ -> [_ _ _ _ _ _ _ _ _ _ _ _ _ _ _ _ _ _ _ _ _ _ _]
          timeout: 1000 -> [_ _ _ _ _ _ _ _ _ _ _ _ _ _ _ _ _ _ _ _ _ _ _]
          tunnel: w85 -> [_ _ w89 _ w171 w216 _ w301 w336 w356 _ _ w436 _ w500 _ _ _ _ _ _ _ w644]
          tunnel: w83 -> [_ _ _ _ _ _ _ _ _ _ _ _ _ _ _ _ _ _ _ _ _ _ _]
          event Timeout {
            n72 = event-data() -> ()  [unwired: 3 out]
            n73 = property on="Waiting" class="Str"("Visible"=FALSE) -> ()  [unwired: 2 in, 2 out]
          }
          event "Save Sample Information": Value Change {
            # "should trigger this when ever a new session is created."
            n74 = event-data() -> ()  [unwired: 7 out]
            n75 = local write "Save Sample Information"(FALSE ("Save")) -> ()
          }
          event "Load": Value Change {
            # "if cancel\ndon't do anything"
            n76 = event-data() -> ("CtlRef"=w92:refnum<vi>)  [unwired: 6 out]
            n77 = local read "Sample_data_base"() -> (w95:path)
            n78 = property class="Bool (strict)"(reference=w92, "Value"=FALSE) -> ()  [unwired: 1 in, 2 out]
            n79 = call "File Dialog"("start path"=w95, "prompt"="Select file for the\nsample data base", "pattern (all files)"="*.xml") -> ("selected path"=w97:path, "cancelled"=w96:bool, "error out"=w90:errorcluster)  [unwired: 9 in, 1 out]
            n80 = local write "error out 3"(w90) -> ()
            n81 = case shown="False" w96 {
              tunnel: w89 -> [w120 _]
              tunnel: w97 -> [w109 _]
              frame False {
                w101 = T10."Enabled" ("Disabled")
                # "Things done here:\n1. prompt user to select the main data base file.\n2. read it and adjust format of file paths as appropriate for Macs or PCs\n3. Sets variable Sample_data_base with the file path to the main data base\n4. Creates the table of spots versus sessions\n5. Grays out or enables add, transform, etc based on number of spots and\n    number of sessions\n6. loads the last session in the data base as the current session\n7. if there are enough fiducials in the current session calculate the\n     transform and move all spots from the previous session forward\n     cascade through in case there is an old sample data base that\n     hasn't done this.\n8. load up the sessions for this sample drop down\n9. put a value into sample information and signal it so that event gets \n     called."
                # "load should make the last session for this sample the current session by default.\nIf sample was removed from the machine a new session should be started."
                n82 = local write "Sample_data_base"(w109) -> ()
                n83 = property on="Start New Session" class="Bool (strict)"("DisabledEnum"=w101) -> ()  [unwired: 2 in, 2 out]
                n84 = property on="Save Sample Information" class="Bool (strict)"("DisabledEnum"=w101) -> ()  [unwired: 2 in, 2 out]
                n85 = property on="Tab Control" class="TabCtl (strict)"("DisabledEnum"=w101) -> ()  [unwired: 2 in, 2 out]
                n86 = local read "Sample Information"() -> (w114:T5)
                n87 = property on="Waiting" class="Str"("Visible"=TRUE) -> (error out=w111:errorcluster)  [unwired: 2 in, 1 out]
                n88 = local write "Tab Control"(T4."Sample Information" ("Tab Control")) -> ()
                n89 = call-poly <vilib>:"Read From XML File.vi"("error in (no error)"=w111, "XML File Path"=w109) -> ("XML Elements"=w117:string)  [unwired: 9 out]
                n90 = call "Correct_Paths_For_OS_in_XML.vi"("XML Elements"=w117) -> ("String"=w116:string)  [unwired: 1 in]
                n91 = Unflatten From XML(xml string=w116, type=w114) -> (value=w110:T5, error out=→"error out 3":errorcluster)  [unwired: 1 in]
                n92 = call "adjust_session_paths.vi"("Sample_Information In"=w110, "top_level"=w109) -> ("MostRecentSessionOut"=w105:T13, "Sample_Information_out"=w108:T12)  [unwired: 1 in]
                n93 = local read "Current Session View"() -> (w106:T1)
                n94 = Unbundle By Name(w105) -> ("Session_data_base"=w104:path)
                n95 = Unbundle By Name(w108) -> ("Session_list"=w107:T14)
                n96 = Array Size(array=w107) -> (size(s)=w98:i32)
                n97 = Bundle By Name(cluster=w106, "CollectionFile"=w104) -> (w103:T1)
                n98 = for {
                  N: w98 -> [_]
                  tunnel: w108 -> [w127]
                  tunnel: w107 -> [w130]
                  tunnel: w109 -> [w128]
                  tunnel: w103 -> [_]
                  i -> [w124]
                  n99 = Decrement(x=w124) -> (x-1=w123:i32)
                  n100 = Index Array(array=w130, index=w124) -> (element=w125:T13)
                  n101 = Unbundle By Name(w125) -> ("Session_data_base"=w129:path)
                  n102 = case shown="True" TRUE {
                    tunnel: w127 -> [_ w144]
                    tunnel: w123 -> [_ w143]
                    tunnel: w129 -> [_ w142]
                    tunnel: w128 -> [_ w140]
                    frame False {
                    }
                    frame True {
                      # "just send in a \nbogus path so this isn't \nchosen"
                      n103 = call "load_current_session.vi"("Current Session Information"=T1 {"CollectionOfPoints"=[], "Instrument"=enum."Unknown", "CollectionFile"=path "kfaj;ldkfja;f", "Session Name/ID"="", "SessionNotes"=""}, "TopLevelDataFilePath"=w140, "just a file"=w142) -> ("Fiducial Count"=w139:u32[], "Sample Set"=w141:T1)  [unwired: 1 in, 1 out]
                      "Sample Set" <- w141
                      n104 = Array Size(array=w139) -> (size(s)=w138:i32)
                      n105 = Greater Or Equal?(x=w138, y=3) -> (x >= y?=w136:bool)
                      n106 = case shown="True" w136 {
                        tunnel: w144 -> [_ w152]
                        tunnel: w143 -> [_ w151]
                        tunnel: w141 -> [w145 w150]
                        tunnel: w140 -> [_ w149]
                        tunnel: [w145 w148] -> w131
                        frame False {
                        }
                        frame True {
                          n107 = call "cm2nm_transform_all_unvarified_spots.vi"("Sample_Information"=w152, "Current Session Information IN"=w150, "ReferenceSessionIndex"=w151, "TopLevelDataFilePath"=w149) -> ("Session Name/ID"=w155:string, "transfomration_matrices"=w147:T7, "FidcucialMetrics"=→"FidcucialMetrics":cluster{"M1":dbl, "M2":dbl, "S1":dbl, "S2":dbl}, "Current Session InformationOUT"=w148:T1, "ReferenceSet"=w153:T1, "PairedFiducialNames"=w154:T9)  [unwired: 1 in, 5 out]
                          n108 = local write "current_transformation_matrices"(w147) -> ()
                          n109 = local write "TransformSession Name/ID"(w155) -> ()
                          n110 = local write "PairedFiducialNames"(w154) -> ()
                          n111 = local write "ReferenceSession"(w153) -> ()
                        }
                      }
                      n112 = call "cm2nm_create_list_of_spots.vi"("Current Session"=w131) -> ("Indices_Experimental_positions"=w133:i32[], "Indices of calculated positions"=w135:i32[], "labels_Experimental_positions"=w134:string[])  [unwired: 1 out]
                      n113 = local write "SpotPrevSessionIndex"(w133) -> ()
                      n114 = local write "Current Session View"(w131) -> ()
                      n115 = local write "SpotPrevCalcIndex"(w135) -> ()
                      n116 = property on="Spots Current Session" class="Ring (strict)"("Strings []"=w134) -> ()  [unwired: 2 in, 2 out]
                      n117 = call "cm2nm_write_session_file.vi"("Session Information"=w131) -> ()  [unwired: 1 out]
                    }
                  }
                }
                n118 = local write "Current Session View"(w103) -> ()
                n119 = Array Size(array=w107) -> (size(s)=w119:i32)
                n120 = Greater Than 0?(x=w119) -> (x > 0?=w118:bool)
                n121 = case shown="False" w118 {
                  tunnel: w109 -> [_ _]
                  tunnel: w108 -> [_ _]
                  tunnel: [FALSE ("Value (Signaling)") w158] -> w102
                  frame False {
                    w157 = T10."Disabled and Grayed Out" ("Disabled")
                    # "might want to querry if they want to \nstart a new session."
                    # "grey out because there is \nno existing session"
                    n122 = property on="Add New Spot To Session" class="Bool (strict)"("DisabledEnum"=w157) -> ()  [unwired: 2 in, 2 out]
                    n123 = property on="Calc Trans" class="Bool (strict)"("DisabledEnum"=w157) -> ()  [unwired: 2 in, 2 out]
                    n124 = property on="LoadSessionIntoCurrent" class="Bool (strict)"("DisabledEnum"=w157) -> ()  [unwired: 2 in, 2 out]
                  }
                  frame True {
                    w158 = TRUE ("Value (Signaling)")
                    n125 = property on="LoadSessionIntoCurrent" class="Bool (strict)"("Val(Sgnl)"=w158) -> ()  [unwired: 2 in, 2 out]
                  }
                }
                n126 = property on="Sample Information" class="Clust (strict)"("Val(Sgnl)"=w108) -> ()  [unwired: 2 in, 2 out]
                n127 = for {
                  tunnel: w107 -> [w122] mode=indexing
                  tunnel: [w121] -> w99 mode=indexing
                  n128 = Unbundle By Name(w122) -> ("Session Name/ID"=w121:string)
                }
                n129 = property on="Sessions Spot calc From" class="Ring (strict)"("Strings []"=w99) -> ()  [unwired: 2 in, 2 out]
                n130 = property on="Sessions Spot Transform" class="Ring (strict)"("Strings []"=w99) -> ()  [unwired: 2 in, 2 out]
                n131 = property on="Sessions For This Sample." class="Ring (strict)"("Strings []"=w99) -> (error out=w113:errorcluster)  [unwired: 2 in, 1 out]
                n132 = stacked-sequence {
                  tunnel: w108 -> [_ w162]
                  tunnel: w120 -> [_ w163]
                  tunnel: [_ w163] -> _
                  tunnel: [_ w162] -> _
                  tunnel: w109 -> [_ w161]
                  tunnel: w113 -> [_ _]
                  tunnel: w102 -> [_ _]
                  frame #0 {
                    n133 = local read "Sample Information"() -> (w160:T5)
                    n134 = local read "Sample_data_base"() -> (w159:path)
                    n135 = call "cm2nm_save_sample_information.vi"("Sample_Information"=w160, "Sample_data_base"=w159) -> ()  [unwired: 1 out]
                  }
                  frame #1 {
                    n136 = call "cm2nm_Init_table_on_sampleInfo.vi"("Sample_Information"=w162, "Sample locations of Interest"=w163, "TopLevelDataFilePath"=w161) -> ()  [unwired: 3 out]
                  }
                }
              }
              frame True {
              }
            }
          }
          event Value Change {
            # "cause this event to get a save. Left this here so I could simplify \nbut have just put this routine every where we'd like it to get\nsaved."
            n137 = event-data() -> ()  [unwired: 7 out]
            n138 = local read "Current Session View"() -> (w164:T1)
            n139 = call "cm2nm_write_session_file.vi"("Session Information"=w164) -> ()  [unwired: 1 out]
          }
          event "New Sample": Value Change {
            n140 = event-data() -> ()  [unwired: 7 out]
            n141 = local read "Data Base Directory"() -> (w170:path)
            n142 = local write "New Sample"(FALSE ("New Sample")) -> ()
            n143 = call "New_Sample_dialog.vi"("Base Bath In"=w170) -> ("Notes About this Sample Out"=w168:string, "Sample_name_out"=w169:string, "Sample_data_base"=w166:path, "Cancelled?"=w167:bool, "Base Bath Out"=w165:path)  [unwired: 6 in]
            n144 = case shown="False" w167 {
              tunnel: w171 -> [w193 _]
              tunnel: w167 -> [w192 _]
              tunnel: w169 -> [w191 _]
              tunnel: w168 -> [w190 _]
              tunnel: w166 -> [w183 _]
              tunnel: w165 -> [w177 _]
              frame False {
                w174 = T10."Enabled" ("Disabled")
                w173 = string[] [] ("Strings []")
                w186 = T10."Disabled and Grayed Out" ("Disabled")
                w194 = string[] [] ("Column Header Strings[]")
                # "keep the base directory"
                # "save the old \ndata base"
                # "Reset the Table"
                n145 = local write "Sample_data_base"(w183) -> ()
                n146 = property on="Sessions Spot calc From" class="Ring (strict)"("Strings []"=w173) -> ()  [unwired: 2 in, 2 out]
                n147 = local write "Data Base Directory"(w177) -> ()
                n148 = property on="Sessions For This Sample." class="Ring (strict)"("Strings []"=w173) -> ()  [unwired: 2 in, 2 out]
                n149 = property on="Spots Current Session" class="Ring (strict)"("Strings []"=w173) -> ()  [unwired: 2 in, 2 out]
                n150 = property on="Spots For Selected Session" class="Ring (strict)"("Strings []"=w173) -> ()  [unwired: 2 in, 2 out]
                n151 = property on="Start New Session" class="Bool (strict)"("DisabledEnum"=w174) -> ()  [unwired: 2 in, 2 out]
                n152 = property on="Sessions Spot Transform" class="Ring (strict)"("Strings []"=w173) -> ()  [unwired: 2 in, 2 out]
                n153 = property on="Tab Control" class="TabCtl (strict)"("DisabledEnum"=w174) -> ()  [unwired: 2 in, 2 out]
                n154 = property on="Add New Spot To Session" class="Bool (strict)"("DisabledEnum"=w186) -> ()  [unwired: 2 in, 2 out]
                n155 = property on="Calc Trans" class="Bool (strict)"("DisabledEnum"=w186) -> ()  [unwired: 2 in, 2 out]
                n156 = property on="LoadSessionIntoCurrent" class="Bool (strict)"("DisabledEnum"=w186) -> ()  [unwired: 2 in, 2 out]
                n157 = local read "Sample Information"() -> (w189:T5)
                n158 = local read "Sample_data_base"() -> (w187:path)
                n159 = Bundle By Name(cluster=T11 {"CollectionOfPoints"=[], "Instrument"=0, "CollectionFile"=path "<Not A Path>", "Session Name/ID"="", "SessionNotes"=""} ("Sample Set"), "CollectionFile"=path "") -> (w185:T11)
                n160 = local read "Current Session View"() -> (w182:T1)
                n161 = call "cm2nm_save_sample_information.vi"("Sample_Information"=w189, "Sample_data_base"=w187) -> ("Sample_data_base 2"=w188:path)
                n162 = call "cm2nm_write_session_file.vi"("Session Information"=w182) -> ("NaN/Path/Refnum?"=w181:bool)
                n163 = local write "Sample locations of Interest"(string[][] [] ("Sample locations of Interest")) -> ()
                n164 = local write "Fiducial Count"(u32[] [] ("Fiducial Count")) -> ()
                n165 = case shown="False" w192 {
                  tunnel: w185 -> [w198 _]
                  tunnel: T12 {"Sample Name/ID"="", "Notes on Sample"="", "Session_list"=[]} ("Sample_Information") -> [w203 _]
                  tunnel: w191 -> [w201 _]
                  tunnel: w190 -> [w200 _]
                  tunnel: w188 -> [_ _]
                  tunnel: w181 -> [_ _]
                  frame False {
                    # "start a new session"
                    n166 = local write "Session Information View"(w198) -> ()
                    n167 = local write "Current Session View"(w198) -> ()
                    n168 = Bundle By Name(cluster=w203, "Sample Name/ID"=w201, "Notes on Sample"=w200) -> (w202:T12)
                    n169 = local write "Sample Information"(w202) -> ()
                    n170 = property on="Start New Session" class="Bool (strict)"("Val(Sgnl)"=TRUE ("Value (Signaling)")) -> ()  [unwired: 2 in, 2 out]
                  }
                  frame True {
                  }
                }
                n171 = property on="Add New Spot To Session" class="Bool (strict)"("DisabledEnum"=T10."Disabled and Grayed Out" ("Disabled"), "TipStrip"="Start a new Session before adding spots" ("Tip Strip")) -> ()  [unwired: 2 in, 2 out]
                n172 = property on="Add Fiducial" class="Bool (strict)"("DisabledEnum"=T10."Disabled and Grayed Out" ("Disabled"), "TipStrip"="Start a new Session before adding spots" ("Tip Strip")) -> ()  [unwired: 2 in, 2 out]
                n173 = property on="Property Node" class="Tbl (strict)"(reference=w193, "Column Headers[]"=w194, "Row Headers[]"=w194) -> ()  [unwired: 1 in, 2 out]
              }
              frame True {
              }
            }
          }
          event "Add New Spot To Session", "Add Fiducial": Value Change {
            # "Respond to the add sample buton take the\ninfomration in the new sample form put it in the\narray table and update the fiducial indicator."
            n174 = event-data() -> ("CtlRef"=w211:refnum<vi>)  [unwired: 6 out]
            n175 = property class="Bool (strict)"(reference=w211, "Value"=FALSE) -> ("Label.Text"=w209:string)  [unwired: 1 in, 2 out]
            n176 = local read "Current Session View"() -> (w207:T1)
            n177 = property on="Sample locations of Interest" class="Tbl (strict)"() -> ("Row Headers[]"=w213:string[])  [unwired: 2 in, 2 out]
            n178 = Equal?(x=w209, y="Add Fiducial") -> (x = y?=w204:bool)
            n179 = call "cm2nm_maintain_form_values.vi"("Fiducial"=w204, "Current Session Information"=w207) -> ("Cluster"=w206:T2)
            n180 = call "Add_spot_dialog.vi"("Modify"=FALSE, "TransformedPt"=FALSE, "ArrayOfPointNames"=w213, "CurrentSessionInformation_IN"=w207, "PointInformation_IN"=w206) -> ("PointInformationOut"=w214:T2, "Cancel_OUT"=w215:bool)  [unwired: 4 in, 1 out]
            n181 = case shown="False" w215 {
              tunnel: w216 -> [w229 _]
              tunnel: w214 -> [w238 _]
              frame False {
                w245 = refnum<vi> refnum  # Array
                # "enable buttons based on number of fiducials.\nAlso trigger find all spots in previous session"
                n182 = local read "Sample Information"() -> (w236:T5)
                n183 = local read "Current Session View"() -> (w224:T1)
                n184 = control-ref of="Current Session View"() -> (w242:refnum<vi>)
                n185 = Unbundle By Name(w236) -> ("Session_list"=w221:T6[])
                n186 = call "cm2nm_add_new_sample_point_to_session_array.vi"("Sample Set"=w224, "Enter New Point"=w238) -> ("NewPoint"=w243:T2, "SetIndexOfarrytoEnd"=w241:i32[], "Sample Set Out"=w220:T1, "Fiducial Count"=w235:u32[])  [unwired: 1 in, 2 out]
                n187 = property on="Property Node" class="Clust (strict)"(reference=w242) -> ("Controls[]"=w247:refnum<vi>[])  [unwired: 1 in, 2 out]
                n188 = Unbundle By Name(w220) -> ("CollectionOfPoints"=w223:T2[])
                n189 = local write "Enter New Location/Position"(w243) -> ()
                n190 = local write "Current Session View"(w220) -> ()
                n191 = Array Size(array=w235) -> (size(s)=w237:i32)
                n192 = Array Size(array=w221) -> (size(s)=w232:i32)
                n193 = Decrement(x=w232) -> (x-1=w222:i32)
                n194 = call "cm2nm_add_point_to_list.vi"("SampleDataPoint"=w238, "SessionIndex"=w222, "Sample locations of Interest"=w229) -> ()  [unwired: 1 out]
                n195 = Index Array(array=w247, index=0) -> (element=w240:refnum<vi>)
                n196 = call "cm2nm_write_session_file.vi"("Session Information"=w220) -> ()  [unwired: 1 out]
                n197 = To More Specific Class(target class=w245, reference=w240) -> (specific class reference=w244:refnum<vi>, error out=w230:errorcluster)  [unwired: 1 in]
                n198 = call "Determine_if_transformation is possible.vi"("NUmber of Sessions Prior to Current"=w222, "Session_list"=w221, "numberFidsCurrentSession"=w237, "CollectionOfPoints"=w223) -> ("Fiducial count"=w217:u32[], "AtLeast3MatchingFids"=w219:bool)  [unwired: 6 in]
                n199 = local write "Fiducial Count"(w217) -> ()
                n200 = property class="Arr"(reference=w244, error in=w230, "Index Values"=w241) -> (error out=w231:errorcluster)  [unwired: 1 out]
                n201 = case shown="True" w219 {
                  tunnel: [T10."Disabled and Grayed Out" ("Disabled") T10."Enabled" ("Disabled")] -> w218
                  frame False {
                  }
                  frame True {
                    n202 = property on="FindAllSpotsFromPrevSession" class="Bool (strict)"("Val(Sgnl)"=TRUE ("Value (Signaling)")) -> ()  [unwired: 2 in, 2 out]
                  }
                }
                n203 = Unbundle By Name(w220) -> ("CollectionOfPoints"=w234:T2[])
                n204 = call "cm2nm_create_list_of_spots.vi"("Current Session"=w220) -> ("Indices_Experimental_positions"=w226:i32[], "Indices of calculated positions"=w228:i32[], "labels_Experimental_positions"=w227:string[])  [unwired: 1 out]
                n205 = property on="Spots Current Session" class="Ring (strict)"("Strings []"=w227) -> ()  [unwired: 2 in, 2 out]
                n206 = local write "SpotPrevSessionIndex"(w226) -> ()
                n207 = local write "SpotPrevCalcIndex"(w228) -> ()
                n208 = Array Size(array=w234) -> (size(s)=w233:i32)
                n209 = property class="Ctl"(reference=w240, error in=w231) -> ("Label.Text"=→"Label.Text":string)  [unwired: 2 out]
                n210 = case shown="0" w233 {
                  tunnel: [T10."Disabled and Grayed Out" ("Disabled") T10."Enabled" ("Disabled")] -> w225
                  frame 0 {
                  }
                  frame 1, Default {
                  }
                }
                n211 = property on="Transform a Pnt." class="Bool (strict)"("Disabled"=w218) -> ()  [unwired: 2 in, 2 out]
                n212 = property on="Calc Trans" class="Bool (strict)"("Disabled"=w218) -> ()  [unwired: 2 in, 2 out]
                n213 = property on="modify" class="Bool (strict)"("DisabledEnum"=w225) -> ()  [unwired: 2 in, 2 out]
              }
              frame True {
              }
            }
          }
          event "Calc Trans": Value Change {
            n214 = event-data() -> ("CtlRef"=w259:refnum<vi>)  [unwired: 6 out]
            n215 = property class="Bool (strict)"(reference=w259, "Value"=FALSE ("Calc Trans")) -> ()  [unwired: 1 in, 2 out]
            n216 = local read "Sample_data_base"() -> (w254:path)
            n217 = property on="Sample locations of Interest" class="Tbl (strict)"() -> ("Row Headers[]"=w260:string[])  [unwired: 2 in, 2 out]
            n218 = local read "Sample Information"() -> (w255:T5)
            n219 = local read "CurrentRefSessionIdx"() -> (w253:i32)
            n220 = local read "Current Session View"() -> (w257:T1)
            n221 = call "Select spot to transform.vi"("TopLevelDataFilePath"=w254, "Sample Information"=w255, "Current Session Information"=w257, "RefernceSessionInput"=w253) -> ("SelectedSpotInfo"=w261:T2, "Cancel out"=w256:bool)  [unwired: 1 in]
            n222 = case shown="False" w256 {
              tunnel: w261 -> [w263 _]
              tunnel: w260 -> [w267 _]
              tunnel: w257 -> [w265 _]
              tunnel: w255 -> [w262 _]
              frame False {
                n223 = call "Add_spot_dialog.vi"("Modify"=TRUE, "TransformedPt"=TRUE, "ArrayOfPointNames"=w267, "CurrentSessionInformation_IN"=w265, "PointInformation_IN"=w263) -> ("PointInformationOut"=w270:T2, "CurrentSessionInformationOut"=w266:T1, "Cancel_OUT"=w264:bool)  [unwired: 4 in]
                n224 = case shown="False" w264 {
                  tunnel: w270 -> [w288 _]
                  tunnel: w266 -> [w277 _]
                  tunnel: w262 -> [w278 _]
                  frame False {
                    # "make sure\nit gets written\nbefore  it gets\nread here."
                    n225 = call "cm2nm_update_fiducial_indicator.vi"("Sample Set"=w277) -> ("Array"=w280:u32[])
                    n226 = Unbundle By Name(w277) -> ("CollectionOfPoints"=w276:T2[])
                    n227 = Unbundle By Name(w278) -> ("Session_list"=w275:T6[])
                    n228 = local read "Sample Information"() -> (w287:T5)
                    n229 = Array Size(array=w280) -> (size(s)=w279:i32)
                    n230 = local write "Current Session View"(w277) -> ()
                    n231 = call "cm2nm_write_session_file.vi"("Session Information"=w277) -> ("NaN/Path/Refnum?"=w284:bool)
                    n232 = Array Size(array=w275) -> (size(s)=w274:i32)
                    n233 = Unbundle By Name(w287) -> ("Session_list"=w286:T6[])
                    n234 = Decrement(x=w274) -> (x-1=w273:i32)
                    n235 = call "Determine_if_transformation is possible.vi"("NUmber of Sessions Prior to Current"=w273, "Session_list"=w275, "numberFidsCurrentSession"=w279, "CollectionOfPoints"=w276) -> ("Fiducial count"=w272:u32[])  [unwired: 6 in, 1 out]
                    n236 = control-ref of="Sample locations of Interest"() -> (w271:refnum<vi>)
                    n237 = Array Size(array=w286) -> (size(s)=w289:i32)
                    n238 = Decrement(x=w289) -> (x-1=w285:i32)
                    n239 = local write "Fiducial Count"(w272) -> ()
                    n240 = flat-sequence {
                      tunnel: w288 -> [w293]
                      tunnel: w271 -> [w292]
                      tunnel: w285 -> [w291]
                      tunnel: w284 -> [_]
                      frame #0 {
                        # "trigger to recalc\nin case this was\na fiducial"
                        n241 = call "cm2nm_add_point_to_list.vi"("SampleDataPoint"=w293, "SessionIndex"=w291, "Sample locations of Interest"=w292) -> ()  [unwired: 1 out]
                        n242 = property on="FindAllSpotsFromPrevSession" class="Bool (strict)"("Val(Sgnl)"=TRUE ("Value (Signaling)")) -> ()  [unwired: 2 in, 2 out]
                      }
                    }
                    n243 = call "cm2nm_create_list_of_spots.vi"("Current Session"=w277) -> ("Indices_Experimental_positions"=w281:i32[], "Indices of calculated positions"=w283:i32[], "labels_Experimental_positions"=w282:string[])  [unwired: 1 out]
                    n244 = local write "SpotPrevSessionIndex"(w281) -> ()
                    n245 = local write "SpotPrevCalcIndex"(w283) -> ()
                    n246 = property on="Spots Current Session" class="Ring (strict)"("Strings []"=w282) -> ()  [unwired: 2 in, 2 out]
                  }
                  frame True {
                  }
                }
              }
              frame True {
              }
            }
          }
          event "FindAllSpotsFromPrevSession": Value Change {
            # "write out point information in comma delimitted pattern"
            # "reset this to the default of\nfinding the most recent\nprevious session.\n\nthe transform from previous\nsession code now can set\nit."
            n247 = event-data() -> ()  [unwired: 7 out]
            n248 = property on="Waiting" class="Str"("Visible"=TRUE) -> (error out=w299:errorcluster)  [unwired: 2 in, 1 out]
            n249 = stacked-sequence {
              tunnel: w301 -> [w316]
              tunnel: w299 -> [_]
              tunnel: [w310] -> w298
              tunnel: [-1 ("SessionIndex")] -> w294
              frame #0 {
                # "-1 indicates\nto go one session back from the current session"
                n250 = local read "Sample_data_base"() -> (w317:path)
                n251 = local read "Current Session View"() -> (w320:T1)
                n252 = local read "Sample Information"() -> (w315:T5)
                n253 = call "cm2nm_transform_all_unvarified_spots.vi"("Sample_Information"=w315, "Current Session Information IN"=w320, "ReferenceSessionIndex"="SessionIndex", "TopLevelDataFilePath"=w317) -> ("Session Name/ID"=w323:string, "transfomration_matrices"=w306:T7, "CurrentSessionOut"=→"CurrentSessionOut":T2[], "CurrentRefSessionIdx"=→"CurrentRefSessionIdx":i32, "Current Session InformationOUT"=w310:T1, "ReferenceSet"=w321:T1, "Array"=→"Array":bool[], "PairedFiducialNames"=w322:T9)  [unwired: 1 in, 3 out]
                n254 = local write "TransformSession Name/ID"(w323) -> ()
                n255 = local write "Current Session View"(w310) -> ()
                n256 = local write "ReferenceSession"(w321) -> ()
                n257 = local write "PairedFiducialNames"(w322) -> ()
                n258 = call "cm2nm_write_session_file.vi"("Session Information"=w310) -> ("NaN/Path/Refnum?"=w311:bool)
                n259 = stacked-sequence {
                  tunnel: w317 -> [w326]
                  tunnel: w316 -> [w325]
                  tunnel: w315 -> [w324]
                  tunnel: w311 -> [_]
                  frame #0 {
                    n260 = call "cm2nm_Init_table_on_sampleInfo.vi"("Sample_Information"=w324, "Sample locations of Interest"=w325, "TopLevelDataFilePath"=w326) -> ()  [unwired: 3 out]
                  }
                }
                n261 = local write "current_transformation_matrices"(w306) -> ()
                n262 = call "cm2nm_create_list_of_spots.vi"("Current Session"=w310) -> ("Indices_Experimental_positions"=w312:i32[], "Indices of calculated positions"=w314:i32[], "labels_Experimental_positions"=w313:string[])  [unwired: 1 out]
                n263 = local write "SpotPrevCalcIndex"(w314) -> ()
                n264 = local write "SpotPrevSessionIndex"(w312) -> ()
                n265 = property on="Spots Current Session" class="Ring (strict)"("Strings []"=w313) -> ()  [unwired: 2 in, 2 out]
              }
            }
            n266 = local write "FindAllSpotsFromPrevSession"(FALSE ("FindAllSpotsFromPrevSession")) -> ()
            n267 = Unbundle By Name(w298) -> ("CollectionOfPoints"=w297:T2[])
            n268 = for {
              tunnel: w297 -> [w305] mode=indexing
              shift-right: [w304] -> w295
              shift-left: "" ("String Out") -> [w303]
              n269 = call "Print_a_spot.vi"("Position"=w305, "String In"=w303) -> ("String Out"=w304:string)
            }
            "Current_Session_points" <- w295
            n270 = local write "SessionIndex"(w294) -> ()
          }
          event "Transform a Pnt.": Value Change {
            w339 = TRUE  # From a transformed spot. Don't prompt that  it is a repeat since name must  match
            # "This event may be deprecated.  leaving it incase we want the option to re-transform a spot that has been confirmed."
            n271 = event-data() -> ()  [unwired: 7 out]
            n272 = local read "current_transformation_matrices"() -> (w330:T7)
            n273 = local read "Spots Current Session"() -> (w334:u16)
            n274 = property on="Sample locations of Interest" class="Tbl (strict)"() -> ("Row Headers[]"=w340:string[])  [unwired: 2 in, 2 out]
            n275 = local read "Current Session View"() -> (w341:T1)
            n276 = local read "Sample_data_base"() -> (w333:path)
            n277 = local read "Enter New Location/Position"() -> (w343:T2)
            n278 = Unbundle By Name(w330) -> ("A"=w329:T8, "B"=w327:T8, "C"=w328:T8)
            n279 = local read "Sample Information"() -> (w335:T5)
            n280 = local write "Transform a Pnt."(FALSE ("Transform a Pnt.")) -> ()
            n281 = call "cm2nm_transform_reference_location.vi"("Sample locations of Interest"=w336, "Sample_Information"=w335, "TransformReferenceSessionIndex"=w334, "A - Transformation Matrix"=w329, "Enter New Point IN"=w343, "C"=w328, "B - vector offset"=w327, "TopLevelDataFilePath"=w333) -> ("Enter New Point OUT"=w342:T2)
            n282 = local write "Enter New Location/Position"(w342) -> ()
            n283 = call "Add_spot_dialog.vi"("Modify"=TRUE, "TransformedPt"=w339, "ArrayOfPointNames"=w340, "CurrentSessionInformation_IN"=w341, "PointInformation_IN"=w342) -> ("PointInformationOut"=w337:T2, "CurrentSessionInformationOut"=w338:T1, "Cancel_OUT"=w332:bool)  [unwired: 4 in]
            n284 = case shown="False" w332 {
              tunnel: w338 -> [w345 _]
              tunnel: w337 -> [w352 _]
              tunnel: w336 -> [w351 _]
              tunnel: w335 -> [w350 _]
              frame False {
                # "send in the last session index\nwhich is the current session\nas well."
                n285 = Unbundle By Name(w350) -> ("Session_list"=w349:T6[])
                n286 = call "cm2nm_write_session_file.vi"("Session Information"=w345) -> ()  [unwired: 1 out]
                n287 = call "cm2nm_update_fiducial_indicator.vi"("Sample Set"=w345) -> ("Array"=w355:u32[])
                n288 = local write "Current Session View"(w345) -> ()
                n289 = call "cm2nm_create_list_of_spots.vi"("Current Session"=w345) -> ("Indices_Experimental_positions"=w346:i32[], "Indices of calculated positions"=w348:i32[], "labels_Experimental_positions"=w347:string[])  [unwired: 1 out]
                n290 = local write "Fiducial Count"(w355) -> ()
                n291 = Array Size(array=w349) -> (size(s)=w354:i32)
                n292 = local write "SpotPrevCalcIndex"(w348) -> ()
                n293 = local write "SpotPrevSessionIndex"(w346) -> ()
                n294 = property on="Spots Current Session" class="Ring (strict)"("Strings []"=w347) -> ()  [unwired: 2 in, 2 out]
                n295 = Decrement(x=w354) -> (x-1=w353:i32)
                n296 = call "cm2nm_add_point_to_list.vi"("SampleDataPoint"=w352, "SessionIndex"=w353, "Sample locations of Interest"=w351) -> ()  [unwired: 1 out]
              }
              frame True {
              }
            }
          }
          event "modify": Value Change {
            n297 = event-data() -> ("CtlRef"=w370:refnum<vi>, "OldVal"=w369:bool)  [unwired: 5 out]
            n298 = property class="Bool (strict)"(reference=w370, "Value"=w369) -> ()  [unwired: 1 in, 2 out]
            n299 = local read "Current Session View"() -> (w359:T1)
            n300 = property on="Sample locations of Interest" class="Tbl (strict)"() -> ("Row Headers[]"=w364:string[])  [unwired: 2 in, 2 out]
            n301 = local read "Spots Current Session"() -> (w361:u16)
            n302 = Unbundle By Name(w359) -> ("CollectionOfPoints"=w357:T2[])
            n303 = local read "SpotPrevSessionIndex"() -> (w360:i32[])
            n304 = Index Array(array=w360, index=w361) -> (element=w358:i32)
            n305 = Index Array(array=w357, index=w358) -> (element=w367:T2)
            n306 = call "Add_spot_dialog.vi"("Modify"=TRUE, "TransformedPt"=FALSE, "ArrayOfPointNames"=w364, "CurrentSessionInformation_IN"=w359, "PointInformation_IN"=w367) -> ("PointInformationOut"=w368:T2, "CurrentSessionInformationOut"=w363:T1, "Cancel_OUT"=w362:bool)  [unwired: 4 in]
            n307 = case shown="False" w362 {
              tunnel: w368 -> [w379 _]
              tunnel: w356 -> [w387 _]
              tunnel: w363 -> [_ _]
              tunnel: w359 -> [w383 _]
              tunnel: w358 -> [w380 _]
              tunnel: w357 -> [w381 _]
              frame False {
                # "replace it in the array\nhere."
                # "send in the last session index\nwhich is the current session\nas well."
                n308 = Replace Array Subset(array=w381, new element=w379, index=w380) -> (w378:T2[])
                n309 = Bundle By Name(cluster=w383, "CollectionOfPoints"=w378) -> (w382:T1)
                n310 = local write "Current Session View"(w382) -> ()
                n311 = local read "Sample Information"() -> (w389:T5)
                n312 = call "cm2nm_create_list_of_spots.vi"("Current Session"=w382) -> ("Indices_Experimental_positions"=w384:i32[], "Indices of calculated positions"=w386:i32[], "labels_Experimental_positions"=w385:string[])  [unwired: 1 out]
                n313 = local write "SpotPrevSessionIndex"(w384) -> ()
                n314 = local write "SpotPrevCalcIndex"(w386) -> ()
                n315 = Unbundle By Name(w389) -> ("Session_list"=w388:T6[])
                n316 = property on="Spots Current Session" class="Ring (strict)"("Strings []"=w385) -> ()  [unwired: 2 in, 2 out]
                n317 = call "cm2nm_update_fiducial_indicator.vi"("Sample Set"=w382) -> ("Array"=w377:u32[])
                n318 = call "cm2nm_write_session_file.vi"("Session Information"=w382) -> ()  [unwired: 1 out]
                n319 = Array Size(array=w388) -> (size(s)=w390:i32)
                n320 = Array Size(array=w377) -> (size(s)=w376:i32)
                n321 = local write "Fiducial Count"(w377) -> ()
                n322 = Greater Or Equal?(x=w376, y=3) -> (x >= y?=w373:bool)
                n323 = Decrement(x=w390) -> (x-1=w374:i32)
                n324 = Greater Than 0?(x=w374) -> (x > 0?=w372:bool)
                n325 = call "cm2nm_add_point_to_list.vi"("SampleDataPoint"=w379, "SessionIndex"=w374, "Sample locations of Interest"=w387) -> ()  [unwired: 1 out]
                n326 = And(x=w372, y=w373) -> (x .and. y?=w371:bool)
                n327 = case shown="True" w371 {
                  frame False {
                  }
                  frame True {
                    n328 = property on="FindAllSpotsFromPrevSession" class="Bool (strict)"("Val(Sgnl)"=TRUE ("Value (Signaling)")) -> ()  [unwired: 2 in, 2 out]
                  }
                }
              }
              frame True {
                # "if the action is canceled nothing to do"
              }
            }
          }
          event "Edit Spot": Value Change {
            # "Get data from selected spot and allow the user to modify the information\nCurrently I will not restrict any modifications But probably should At least\nname."
            n329 = event-data() -> ("CtlRef"=w399:refnum<vi>, "OldVal"=w398:bool)  [unwired: 5 out]
            n330 = local read "Sample Information"() -> (w397:T5)
            n331 = property class="Bool (strict)"(reference=w399, "Value"=w398) -> ()  [unwired: 1 in, 2 out]
            n332 = Unbundle By Name(w397) -> ("Session_list"=w396:T6[])
            n333 = local read "Sessions For This Sample."() -> (w394:u16)
            n334 = Array Size(array=w396) -> (size(s)=w395:i32)
            n335 = Decrement(x=w395) -> (x-1=w393:i32)
            n336 = Less?(x=w394, y=w393) -> (x < y?=w392:bool)
            n337 = case shown="True" w392 {
              tunnel: w394 -> [_ w414]
              tunnel: w396 -> [_ w406]
              frame False {
                n338 = One Button Dialog(message="You have selected a spot in the \ncurrent session. Please click \non the current session tab and\nmodify that spot from there.") -> ()  [unwired: 1 in, 1 out]
              }
              frame True {
                n339 = Index Array(array=w406, index=w414) -> (element=w409:T6)
                n340 = local read "Sample_data_base"() -> (w405:path)
                n341 = Unbundle By Name(w409) -> ("Session_data_base"=w413:path)
                n342 = property on="Sample locations of Interest" class="Tbl (strict)"() -> ("Row Headers[]"=w415:string[])  [unwired: 2 in, 2 out]
                n343 = call "cm2nm_read_session_data_file.vi"("TopLevelDataFilePath"=w405, "Session_data_base"=w413) -> ("Session Information"=w408:T1)  [unwired: 1 in]
                n344 = local read "Spots For Selected Session"() -> (w411:u16)
                n345 = Unbundle By Name(w408) -> ("CollectionOfPoints"=w412:T2[])
                n346 = Index Array(array=w412, index=w411) -> (element=w410:T2)
                n347 = call "Add_spot_dialog.vi"("Modify"=TRUE, "TransformedPt"=FALSE, "ArrayOfPointNames"=w415, "CurrentSessionInformation_IN"=w408, "PointInformation_IN"=w410) -> ("CurrentSessionInformationOut"=w401:T1, "Cancel_OUT"=w407:bool)  [unwired: 4 in, 1 out]
                n348 = case shown="False" w407 {
                  tunnel: w401 -> [w418 _]
                  frame False {
                    n349 = local write "Session Information View"(w418) -> ()
                    n350 = call "cm2nm_write_session_file.vi"("Session Information"=w418) -> ()  [unwired: 1 out]
                  }
                  frame True {
                  }
                }
                n351 = call "cm2nm_create_list_of_spots.vi"("Current Session"=w401) -> ("Indices_Experimental_positions"=w402:i32[], "Indices of calculated positions"=w404:i32[], "labels_Experimental_positions"=w403:string[])  [unwired: 1 out]
                n352 = property on="Spots Current Session" class="Ring (strict)"("Strings []"=w403) -> ()  [unwired: 2 in, 2 out]
                n353 = local write "SpotPrevSessionIndex"(w402) -> ()
                n354 = local write "SpotPrevCalcIndex"(w404) -> ()
              }
            }
          }
          event "Spots Current Session": Value Change {
            w428 = refnum<vi> refnum  # Array
            # "find the collection of points\nfield and set the index to\nthe value passed."
            n355 = event-data() -> ("NewVal"=w420:u16)  [unwired: 6 out]
            n356 = local read "SpotPrevSessionIndex"() -> (w421:i32[])
            n357 = property on="Current Session View" class="Clust (strict)"() -> ("Controls[]"=w430:refnum<vi>[])  [unwired: 2 in, 2 out]
            n358 = for {
              tunnel: w430 -> [w435] mode=indexing
              tunnel: [w431] -> w429
              stop <- w432 stop-if-true
              n359 = property class="Ctl"(reference=w435) -> (reference out=w431:refnum<vi>, "Label.Text"=w434:string)  [unwired: 1 in, 1 out]
              n360 = Equal?(x=w434, y="CollectionOfPoints") -> (x = y?=w432:bool)
            }
            n361 = Index Array(array=w421, index=w420) -> (element=w419:i32)
            n362 = local read "Current Session View"() -> (w425:T1)
            n363 = Build Array(w419) -> (w427:i32[])
            n364 = Unbundle By Name(w425) -> ("CollectionOfPoints"=w424:T2[])
            n365 = To More Specific Class(target class=w428, reference=w429) -> (specific class reference=w426:refnum<vi>)  [unwired: 1 in, 1 out]
            n366 = Index Array(array=w424, index=w419) -> (element=w423:T2)
            n367 = property class="Arr"(reference=w426, "Index Values"=w427) -> ()  [unwired: 1 in, 2 out]
            n368 = Unbundle By Name(w423) -> ("Group"=→"current selection group":i32)
          }
          event "delete": Value Change {
            n369 = event-data() -> ()  [unwired: 7 out]
            n370 = control-ref of="Current Session View"() -> (w437:refnum<vi>)
            n371 = Two Button Dialog(message="Are you sure you want to delete\n the selected Splot", 2:"Yes" ("T button name (\"OK\")")) -> (T button?=w438:bool)  [unwired: 1 out]
            n372 = case shown="True" w438 {
              tunnel: w437 -> [_ w465]
              tunnel: w436 -> [w441 w443]
              tunnel: [w441 w443] -> _
              frame False {
              }
              frame True {
                w469 = refnum<vi> refnum  # Array
                # "Deleting has a bug. Need to delete the X and take it out of the table if\nit's the last session with an X."
                n373 = local read "Sample Information"() -> (w445:T5)
                n374 = property on="Property Node" class="Clust (strict)"(reference=w465) -> ("Controls[]"=w466:refnum<vi>[])  [unwired: 1 in, 2 out]
                n375 = local read "Current Session View"() -> (w459:T1)
                n376 = Unbundle By Name(w445) -> ("Session_list"=w452:T6[])
                n377 = Index Array(array=w466, index=0) -> (element=w468:refnum<vi>)
                n378 = To More Specific Class(target class=w469, reference=w468) -> (specific class reference=w464:refnum<vi>, error out=w463:errorcluster)  [unwired: 1 in]
                n379 = Array Size(array=w452) -> (size(s)=w453:i32)
                n380 = property class="Arr"(reference=w464, error in=w463) -> ("Index Values"=w462:u32[])  [unwired: 2 out]
                n381 = Greater?(x=w453, y=1) -> (0:w451:bool)
                n382 = Index Array(array=w462, index=0) -> (element=w460:u32)
                n383 = call "cm2nm_Delete_sample_location_from_array.vi"("Sample Set In"=w459, "Index2Delete"=w460, "Sample locations of Interest"=w443) -> ("Sample Set Out"=w449:T1)  [unwired: 4 out]
                n384 = local write "Current Session View"(w449) -> ()
                n385 = call "cm2nm_update_fiducial_indicator.vi"("Sample Set"=w449) -> ("Array"=w458:u32[])
                n386 = Array Size(array=w458) -> (size(s)=w455:i32)
                n387 = case shown="3, Default" w455 {
                  tunnel: [w475 T10."Enabled" ("Disabled") w479] -> _
                  tunnel: [w475 T10."Disabled and Grayed Out" ("Disabled") w479] -> w456
                  tunnel: w451 -> [_ _ w478]
                  frame 0 {
                    (unwired) T10."Enabled" ("Disabled")
                    w475 = T10."Disabled and Grayed Out" ("Disabled")
                  }
                  frame 1, 2 {
                  }
                  frame 3, Default {
                    n388 = case shown="False" w478 {
                      tunnel: [T10."Disabled and Grayed Out" ("Disabled") T10."Enabled" ("Disabled")] -> w479
                      frame False {
                      }
                      frame True {
                      }
                    }
                  }
                }
                n389 = local write "Fiducial Count"(w458) -> ()
                n390 = local read "Sample_data_base"() -> (w444:path)
                n391 = call "cm2nm_write_session_file.vi"("Session Information"=w449) -> ()  [unwired: 1 out]
                n392 = property on="Calc Trans" class="Bool (strict)"("Disabled"=w456) -> ()  [unwired: 2 in, 2 out]
                n393 = property on="Transform a Pnt." class="Bool (strict)"("Disabled"=w456) -> ()  [unwired: 2 in, 2 out]
                n394 = stacked-sequence {
                  tunnel: w445 -> [w472]
                  tunnel: [w472] -> _
                  tunnel: w444 -> [w471]
                  tunnel: w443 -> [w470]
                  frame #0 {
                    n395 = call "cm2nm_Init_table_on_sampleInfo.vi"("Sample_Information"=w472, "Sample locations of Interest"=w470, "TopLevelDataFilePath"=w471) -> ()  [unwired: 3 out]
                  }
                }
                n396 = property on="Spots Current Session" class="Ring (strict)"("Val(Sgnl)"=0) -> ()  [unwired: 2 in, 2 out]
                n397 = call "cm2nm_create_list_of_spots.vi"("Current Session"=w449) -> ("Indices_Experimental_positions"=w447:i32[], "Indices of calculated positions"=w448:i32[], "labels_Experimental_positions"=w446:string[])  [unwired: 1 out]
                n398 = Array Size(array=w446) -> (size(s)=w450:i32)
                n399 = case shown="1, Default" w450 {
                  tunnel: [T10."Disabled and Grayed Out" ("Disabled") T10."Enabled" ("Disabled")] -> w442
                  frame 0 {
                  }
                  frame 1, Default {
                  }
                }
                n400 = local write "SpotPrevSessionIndex"(w447) -> ()
                n401 = local write "SpotPrevCalcIndex"(w448) -> ()
                n402 = property on="Spots Current Session" class="Ring (strict)"("Strings []"=w446) -> ()  [unwired: 2 in, 2 out]
                n403 = property on="modify" class="Bool (strict)"("DisabledEnum"=w442) -> ()  [unwired: 2 in, 2 out]
              }
            }
          }
          event "Plot": Value Change {
            n404 = event-data() -> ("CtlRef"=w483:refnum<vi>)  [unwired: 6 out]
            n405 = local read "Current Session View"() -> (w485:T1)
            n406 = Unbundle By Name(w485) -> ("CollectionOfPoints"=w484:T2[])
            n407 = property class="Bool (strict)"(reference=w483, "Value"=FALSE ("Value (Signaling)")) -> ()  [unwired: 1 in, 2 out]
            n408 = call "cm2nm_create_graph_of_session.vi"("CollectionOfSpots"=w484) -> ("X/Y plot array of spots"=→"Spots in Current Session":cluster{dbl[], dbl[]}[])
          }
          event "NewSession_from_previous", "Start New Session": Value Change {
            n409 = event-data() -> ("CtlRef"=w496:refnum<vi>)  [unwired: 6 out]
            n410 = local read "Sample_data_base"() -> (w491:path)
            n411 = local write "Tab Control"(T4."Current Session" ("Tab Control")) -> ()
            n412 = property class="Bool (strict)"(reference=w496, "Value"=FALSE ("Start New Session")) -> ("Label.Text"=w494:string)  [unwired: 1 in, 2 out]
            n413 = Equal?(x=w494, y="NewSession_from_previous") -> (x = y?=w492:bool)
            n414 = case shown="True" w492 {
              tunnel: w491 -> [w508 w514]
              tunnel: [w508 w514] -> w490
              tunnel: [T2[] [] ("CollectionOfPoints") w511] -> w489
              tunnel: [-1 ("SessionIndex") w509] -> w487
              frame False {
              }
              frame True {
                # "mostly debug code. Get selected spots from\na previous session. Also allow for text transforms."
                n415 = local read "Sample Information"() -> (w519:T5)
                n416 = local read "Sessions Spot Transform"() -> (w510:u16)
                n417 = Unbundle By Name(w519) -> ("Session_list"=w518:T6[])
                n418 = Index Array(array=w518, index=w510) -> (element=w517:T6)
                n419 = Unbundle By Name(w517) -> ("Session_data_base"=w516:path)
                n420 = call "load_current_session.vi"("Current Session Information"=T1 {"CollectionOfPoints"=[], "Instrument"=enum."Unknown", "CollectionFile"=path "kfaj;ldkfja;f", "Session Name/ID"="", "SessionNotes"=""}, "TopLevelDataFilePath"=w514, "just a file"=w516) -> ("Sample Set"=w515:T1)  [unwired: 1 in, 2 out]
                n421 = call "Session_from_previous_session_dialog.vi"("Current Session Information"=w515) -> ("Current Session Information Out"=w512:T1)  [unwired: 9 in, 1 out]
                n422 = Unbundle By Name(w512) -> ("CollectionOfPoints"=w511:T2[])
                n423 = local read "Sessions Spot calc From"() -> (w509:u16)
              }
            }
            n424 = local read "Current Session View"() -> (w499:T1)
            n425 = Strip Path(path=w490) -> (stripped path=w497:path)  [unwired: 1 out]
            n426 = call "cm2nm_new_session_dialog.vi"("Session File"=w497) -> ("Session File_out"=w503:path, "Session Name/ID_out"=w502:string, "Notes_out"=w501:string, "Instrument_out"=w504:u16)  [unwired: 3 in, 4 out]
            n427 = call "cm2nm_write_session_file.vi"("Session Information"=w499) -> ("NaN/Path/Refnum?"=w498:bool)
            n428 = Not A Number/Path/Refnum?(number/path/refnum=w503) -> (NaN/Path/Refnum?=w505:bool)
            n429 = case shown="False" w505 {
              tunnel: w504 -> [w544 _]
              tunnel: w503 -> [w543 _]
              tunnel: w502 -> [w533 _]
              tunnel: w501 -> [w542 _]
              tunnel: w500 -> [w540 _]
              tunnel: w498 -> [_ _]
              tunnel: w489 -> [w523 _]
              frame False {
                w531 = T10."Enabled" ("Disabled")
                # "Force a save of sample"
                n430 = local read "Sample Information"() -> (w529:T5)
                n431 = local read "Sample_data_base"() -> (w526:path)
                n432 = property on="LoadSessionIntoCurrent" class="Bool (strict)"("Val(Sgnl)"=TRUE ("Value (Signaling)")) -> ()  [unwired: 2 in, 2 out]
                n433 = property on="Spots Current Session" class="Ring (strict)"("Strings []"=string[] []) -> ()  [unwired: 2 in, 2 out]
                n434 = call "cm2nm_initialize_new_session.vi"("Sample locations of Interest"=w540, "Sample_Information"=w529, "Session File"=w543, "Instrument"=w544, "Session Name/ID"=w533, "Notes_out"=w542) -> ("Sample_out"=w525:T12, "Current Session Information"=w537:T1, "Fiducial Count"=w541:u32[])
                n435 = Unbundle By Name(w525) -> ("Session_list"=w528:T14)
                n436 = call "cm2nm_save_sample_information.vi"("Sample_Information"=w525, "Sample_data_base"=w526) -> ()  [unwired: 1 out]
                n437 = local write "Sample Information"(w525) -> ()
                n438 = local write "Fiducial Count"(w541) -> ()
                n439 = for {
                  tunnel: w528 -> [w546] mode=indexing
                  tunnel: [w545] -> w520 mode=indexing
                  n440 = Unbundle By Name(w546) -> ("Session Name/ID"=w545:string)
                }
                n441 = Bundle By Name(cluster=w537, "CollectionOfPoints"=w523) -> (w524:T1)
                n442 = property on="Sessions For This Sample." class="Ring (strict)"("Strings []"=w520) -> ()  [unwired: 2 in, 2 out]
                n443 = property on="modify" class="Bool (strict)"("DisabledEnum"=T10."Disabled and Grayed Out" ("Disabled")) -> ()  [unwired: 2 in, 2 out]
                n444 = local write "Tab Control"(T4."Current Session" ("Tab Control")) -> ()
                n445 = local write "Current Session View"(w524) -> ()
                n446 = property on="Add New Spot To Session" class="Bool (strict)"("DisabledEnum"=T10."Enabled" ("Disabled"), "TipStrip"="Click to add a new spot to this session." ("Tip Strip")) -> ()  [unwired: 2 in, 2 out]
                n447 = property on="Add Fiducial" class="Bool (strict)"("DisabledEnum"=w531, "TipStrip"="Click to add a new fiducial to this session." ("Tip Strip")) -> ()  [unwired: 2 in, 2 out]
                n448 = property on="Save Sample Information" class="Bool (strict)"("DisabledEnum"=w531) -> ()  [unwired: 2 in, 2 out]
                n449 = property on="Save Sample Information" class="Bool (strict)"("Val(Sgnl)"=TRUE ("Value (Signaling)")) -> ()  [unwired: 2 in, 2 out]
                n450 = call "cm2nm_write_session_file.vi"("Session Information"=w524) -> ()  [unwired: 1 out]
                n451 = property on="Spots Current Session" class="Ring (strict)"("Val(Sgnl)"=0) -> ()  [unwired: 2 in, 2 out]
                n452 = property on="Calc Trans" class="Bool (strict)"("DisabledEnum"=T10."Disabled and Grayed Out" ("Disabled")) -> ()  [unwired: 2 in, 2 out]
                n453 = property on="Sessions Spot Transform" class="Ring (strict)"("Strings []"=w520) -> ()  [unwired: 2 in, 2 out]
                n454 = property on="Sessions Spot calc From" class="Ring (strict)"("Strings []"=w520) -> ()  [unwired: 2 in, 2 out]
              }
              frame True {
                # "if not a path do nothing"
              }
            }
            n455 = local write "SessionIndex"(w487) -> ()
          }
          event Panel Close? {
            n456 = event-data() -> ()  [unwired: 5 out]
            n457 = property on="stop" class="Bool"("Val(Sgnl)"=TRUE ("stop")) -> ()  [unwired: 2 in, 2 out]
            n458 = event-data("Discard?"=TRUE) -> ()  [unwired: 1 in, 1 out]
          }
          event "Batch Add MetaDataFiles": Value Change {
            n459 = event-data() -> ()  [unwired: 7 out]
            n460 = local write "Batch Add MetaDataFiles"(FALSE ("Batch Add MetaDataFiles")) -> ()
            n461 = call "File Dialog3"() -> ()  [unwired: 12 in, 4 out]
          }
          event Value Change; Mouse Down {
            w561 = refnum<vi> refnum  # Array
            # "Happen to know the\narray is element 2 \nof  the cluster. Just the\norder it was made in."
            n462 = event-data() -> ()  [unwired: 5 out]
            n463 = property on="Sample Information" class="Clust (strict)"() -> ("Controls[]"=w564:refnum<vi>[])  [unwired: 2 in, 2 out]
            n464 = Index Array(array=w564, index=2) -> (element=w562:refnum<vi>)
            n465 = local read "Sample Information"() -> (w557:T5)
            n466 = To More Specific Class(target class=w561, reference=w562) -> (specific class reference=w560:refnum<vi>)  [unwired: 1 in, 1 out]
            n467 = property class="Arr"(reference=w560) -> ("Index Values"=w559:u32[])  [unwired: 1 in, 2 out]
            "Index Values" <- w559
            n468 = Unbundle By Name(w557) -> ("Session_list"=w556:T6[])
            n469 = Index Array(array=w559, index=0) -> (element=w555:u32)
            n470 = Array Size(array=w556) -> (size(s)=w554:i32)
            n471 = Less?(x=w555, y=w554) -> (x < y?=w553:bool)
            n472 = local read "Sample_data_base"() -> (w552:path)
            n473 = property on="Waiting" class="Str"("Visible"=TRUE) -> (error out=w550:errorcluster)  [unwired: 2 in, 1 out]
            n474 = case shown="True" w553 {
              tunnel: w556 -> [_ w581]
              tunnel: w555 -> [_ w580]
              tunnel: w552 -> [_ w571]
              tunnel: w550 -> [_ _]
              frame False {
              }
              frame True {
                w575 = refnum<vi> refnum  # Array
                n475 = Index Array(array=w581, index=w580) -> (element=w582:T6)
                n476 = call "cm2nm_read_session_dataFromSesionItem.vi"("TopLevelDataFilePath"=w571, "Sesions"=w582) -> ("Session_OUT"=w579:T1)  [unwired: 1 in]
                n477 = stacked-sequence {
                  tunnel: w579 -> [w586]
                  tunnel: [w586] -> w568
                  frame #0 {
                    n478 = local write "Session Information View"(w586) -> ()
                  }
                }
                n479 = property on="Session Information View" class="Clust (strict)"() -> ("Controls[]"=w573:refnum<vi>[])  [unwired: 2 in, 2 out]
                n480 = Unbundle By Name(w568) -> ("CollectionOfPoints"=w566:T2[])
                n481 = call "Get_cluster_element_by_name.vi"("Label.Text"="CollectionOfPoints", "Controls[]"=w573) -> ("Ctl Refnum"=w576:refnum<vi>)  [unwired: 1 out]
                n482 = To More Specific Class(target class=w575, reference=w576) -> (specific class reference=w577:refnum<vi>)  [unwired: 1 in, 1 out]
                n483 = for {
                  tunnel: w566 -> [w588] mode=indexing
                  tunnel: [w587] -> w569 mode=indexing
                  n484 = Unbundle By Name(w588) -> ("Location Name/ID"=w587:string)
                }
                n485 = for {
                  tunnel: w566 -> [w585] mode=indexing
                  shift-right: [w584] -> w565
                  shift-left: "" ("String Out") -> [w583]
                  n486 = call "Print_a_spot.vi"("Position"=w585, "String In"=w583) -> ("String Out"=w584:string)
                }
                n487 = Build Array(0) -> (w578:i32[])
                n488 = property class="Arr"(reference=w577, "Index Values"=w578) -> (error out=→"error out 4":errorcluster)  [unwired: 1 in, 1 out]
                n489 = property on="Spots For Selected Session" class="Ring (strict)"("Strings []"=w569) -> ()  [unwired: 2 in, 2 out]
                n490 = local write "Selected_Session_spots"(w565) -> ()
              }
            }
          }
          event "LoadSessionIntoCurrent": Value Change {
            n491 = event-data() -> ()  [unwired: 7 out]
            n492 = local read "Sample Information"() -> (w596:T5)
            n493 = local read "Current Session View"() -> (w610:T1)
            n494 = local read "Sample_data_base"() -> (w590:path)
            n495 = Unbundle By Name(w596) -> ("Session_list"=w595:T6[])
            n496 = call "load_current_session.vi"("Current Session Information"=w610, "TopLevelDataFilePath"=w590) -> ("Fiducial Count"=w609:u32[], "Sample Set"=w603:T1)  [unwired: 2 in, 1 out]
            n497 = local write "LoadSessionIntoCurrent"(FALSE ("LoadSessionIntoCurrent")) -> ()
            n498 = local write "Tab Control"(T4."Current Session" ("Tab Control")) -> ()
            n499 = local write "Fiducial Count"(w609) -> ()
            n500 = local write "Current Session View"(w603) -> ()
            n501 = Array Size(array=w595) -> (size(s)=w594:i32)
            n502 = Greater?(x=w594, y=1) -> (0:w591:bool)
            n503 = Array Size(array=w609) -> (size(s)=w608:i32)
            n504 = Greater?(x=w608, y=2) -> (0:w606:bool)
            n505 = And(x=w606, y=w591) -> (x .and. y?=w592:bool)
            n506 = call "cm2nm_create_list_of_spots.vi"("Current Session"=w603) -> ("Indices_Experimental_positions"=w598:i32[], "Indices of calculated positions"=w602:i32[], "labels_Experimental_positions"=w599:string[])  [unwired: 1 out]
            n507 = case shown="True" w592 {
              frame False {
                n508 = property on="Calc Trans" class="Bool (strict)"("DisabledEnum"=T10."Disabled and Grayed Out" ("Disabled")) -> ()  [unwired: 2 in, 2 out]
              }
              frame True {
                n509 = property on="FindAllSpotsFromPrevSession" class="Bool (strict)"("Val(Sgnl)"=TRUE ("Value (Signaling)")) -> ()  [unwired: 2 in, 2 out]
                n510 = property on="Calc Trans" class="Bool (strict)"("DisabledEnum"=T10."Enabled" ("Disabled")) -> ()  [unwired: 2 in, 2 out]
              }
            }
            n511 = property on="Spots Current Session" class="Ring (strict)"("Strings []"=w599) -> ()  [unwired: 2 in, 2 out]
            n512 = local write "SpotPrevSessionIndex"(w598) -> ()
            n513 = local write "SpotPrevCalcIndex"(w602) -> ()
            n514 = Array Size(array=w599) -> (size(s)=w601:i32)
            n515 = Greater Than 0?(x=w601) -> (x > 0?=w600:bool)
            n516 = case shown="False" w600 {
              tunnel: [T10."Disabled and Grayed Out" ("Disabled") T10."Enabled" ("Disabled")] -> w597
              frame False {
              }
              frame True {
              }
            }
            n517 = property on="Add Fiducial" class="Bool (strict)"("DisabledEnum"=T10."Enabled" ("Disabled")) -> ()  [unwired: 2 in, 2 out]
            n518 = property on="Add New Spot To Session" class="Bool (strict)"("DisabledEnum"=T10."Enabled" ("Disabled")) -> ()  [unwired: 2 in, 2 out]
            n519 = property on="modify" class="Bool (strict)"("DisabledEnum"=w597) -> ()  [unwired: 2 in, 2 out]
          }
          event "Sessions For This Sample.": Value Change {
            w625 = refnum<vi> refnum  # Array
            # "just trigger the action for sample information change."
            n520 = event-data() -> ("NewVal"=w623:u16)  [unwired: 6 out]
            n521 = local write "Spots For Selected Session"(0) -> ()
            n522 = property on="Sample Information" class="Clust (strict)"() -> ("Controls[]"=w626:refnum<vi>[])  [unwired: 2 in, 2 out]
            n523 = call "Get_cluster_element_by_name.vi"("Label.Text"="Session_list", "Controls[]"=w626) -> ("Ctl Refnum"=w620:refnum<vi>)  [unwired: 1 out]
            n524 = property class="Ctl"(reference=w620) -> (reference out=w617:refnum<vi>, "Value"=w619:variant)  [unwired: 1 in, 1 out]
            n525 = Build Array(w623) -> (w621:u16[])
            n526 = property class="Ctl"(reference=w617, "Val(Sgnl)"=w619) -> ()  [unwired: 1 in, 2 out]
            n527 = To More Specific Class(target class=w625, reference=w620) -> (specific class reference=w624:refnum<vi>)  [unwired: 1 in, 1 out]
            n528 = property class="Arr"(reference=w624, "Index Values"=w621) -> ()  [unwired: 1 in, 2 out]
          }
          event "Spots For Selected Session": Value Change {
            w633 = refnum<vi> refnum  # Array
            n529 = event-data() -> ("NewVal"=w628:u16)  [unwired: 6 out]
            n530 = property on="Session Information View" class="Clust (strict)"() -> ("Controls[]"=w627:refnum<vi>[])  [unwired: 2 in, 2 out]
            n531 = call "Get_cluster_element_by_name.vi"("Label.Text"="CollectionOfPoints", "Controls[]"=w627) -> ("Ctl Refnum"=w629:refnum<vi>)  [unwired: 1 out]
            n532 = To More Specific Class(target class=w633, reference=w629) -> (specific class reference=w632:refnum<vi>)  [unwired: 1 in, 1 out]
            n533 = Build Array(w628) -> (w630:u16[])
            n534 = property class="Arr"(reference=w632, "Index Values"=w630) -> ()  [unwired: 1 in, 2 out]
          }
          event "Tab Control": Value Change {
            n535 = event-data() -> ("NewVal"=w634:T4)  [unwired: 6 out]
            n536 = case shown="\"Sample Information\"" w634 {
              frame "Sample Information" {
                # "for now just make sure the string list is updated."
                n537 = property on="Sessions For This Sample." class="Ring (strict)"() -> ("NumItems"=w640:u32)  [unwired: 2 in, 2 out]
                n538 = property on="Sessions For This Sample." class="Ring (strict)"() -> ("Value"=w637:u16)  [unwired: 2 in, 2 out]
                n539 = Decrement(x=w640) -> (x-1=w639:u32)
                n540 = Greater?(x=w637, y=w639) -> (0:w638:bool)
                n541 = Select(t=u16 0, s=w638, f=w637) -> (s? t:f=w636:u16)
                n542 = property on="Sessions For This Sample." class="Ring (strict)"("Val(Sgnl)"=w636) -> ()  [unwired: 2 in, 2 out]
              }
              frame "Position/Session Chart", Default {
              }
            }
          }
          event "Create a Report": Value Change {
            n543 = event-data() -> ()  [unwired: 7 out]
            n544 = local read "Sample Information"() -> (w643:T5)
            n545 = local read "Sample_data_base"() -> (w642:path)
            n546 = local write "Create a Report"(FALSE ("Create a Report")) -> ()
            n547 = call "Format_html_report.vi"("Sample Information"=w643, "Sample_data_base"=w642, "Table in"=w644) -> ("String"=→"concatenated string":string)  [unwired: 8 in]
          }
        }
      }
    }
    frame #3 {
    }
  }
  n548 = disable-structure shown="Enabled" {
    frame Disabled {
      n549 = local read "Current Session View"() -> (w647:T1)
      n550 = call "load_current_session.vi"("Current Session Information"=w647) -> ("LocationNamesList"=w646:string[], "Sample Set"=w648:T15)
      n551 = local write "Current Session View"(w648) -> ()
      n552 = property on="Spots For Selected Session" class="Ring (strict)"("Strings []"=w646) -> ()  [unwired: 2 in, 2 out]
    }
    frame Enabled {
    }
  }
